vi "Text control 2 v7.1.vi"() -> ()   [LabVIEW 2019]
panel:
  in  "Tab Control":enum32{"Main", "Other parameters"}(tab)
  in  "Plot sample extrema vs time":bool
  out "Line running":i32
  out "Total lines":i32
  out "Path":path=path "C:/users/rlp38/09Apr2009LTtesting/test2.txt"
  out "I vs Vg":cluster{"Y data in":dbl[], "X data in":dbl[]}[](graph)
  out "Is max":dbl format="%.2e"
  out "Id max":dbl format="%.2e"
  out "Ig max":dbl format="%.2e"
  out "Imax vs time":cluster{"Y data in":dbl[], "X data in":dbl[]}[](graph)
  out "Imin vs time":cluster{"Y data in":dbl[], "X data in":dbl[]}[](graph)
  out "I vs Vd":cluster{"Y data in":dbl[], "X data in":dbl[]}[](graph)
  in  "Script":string="#pulsedstressV d 0.03 20 0 0.5 0.0827 5\n#\n#itime m\n#gaterangemode a\n#drainrangemode a\n#pulsed on 0.05 0 0.02\n#transfer d -10 40 1 5 40 35\n#transfer d -10 40 1 5 40 35\n#transfer d -10 40 1 5 40 35\n#output d 0 40 20 0 40 1\n#\n#\n#sample 1 0.008 221 6 0.003\n#samplei 400e-6 200 6 0.002 0.1\n#vsu2pulse -10 4\n#\n#stressV 0.016 0.03 2e-4 0.1e-3 11\n#stressI 220e-7 0.08 15\n#transfer s -1 1 0.5 -0.005 0.005 0.005\n#output s 0 0 0 -0.008 0.008 0.002"
  out "Command running:":string
  out "Serial port data":string
  out "Elapsed Time":dbl caption="Elapsed Time (s)"
  in  "Time Units":u16(ring)=1 items=["Seconds", "Minutes", "Hours"]
  in  "Time Offset":dbl caption="Set Start Time (s)"
  in  "Reset":bool
  in  "Auto Reset":bool
  in  "integration time":u32(slide) max=2 step=1 scale=0.0..2.0
  out "Is on":dbl format="%.2e"
  out "Id on":dbl format="%.2e"
  out "Ig on":dbl format="%.2e"
  out "Ion vs time":cluster{"Y data in":dbl[], "X data in":dbl[]}[](graph)
  out "Ioff vs time":cluster{"Y data in":dbl[], "X data in":dbl[]}[](graph)
  out "Ig min":dbl format="%.2e"
  out "Id min":dbl format="%.2e"
  out "Is min":dbl format="%.2e"
  out "Is off":dbl format="%.2e"
  out "Id off":dbl format="%.2e"
  out "Ig off":dbl format="%.2e"
  in  "Integration time (long)":dbl=0.32 min=0.04 max=2.0 step=0.02 format="%.2f"
  in  "Integration time (short)":dbl=0.0019 min=8e-05 max=0.0019 step=8e-05 format="%^.0e"
  in  "Drain: Compliance":dbl=0.001 format="%.8f"
  in  "Gate: Compliance":dbl=0.001 format="%.8f"
  in  "Interrupt scan":bool
  in  "Interrupt program":bool
  in  "Plot output curve extrema vs time":bool
  in  "Plot transfer curve extrema vs time":bool
  out "I vs time (Bias Stress)":cluster{"Y data in":dbl[], "X data in":dbl[]}[](graph)
  in  "Sample I - Probe 4 (Disabled)":u32(ring)=3 items=["SMU1  ", "SMU2  ", "SMU3  ", "SMU4  ", "SMU5  ", "SMU6  ", "VSU1  ", "VSU2  "]
  in  "Sample I - Source/Common":u32(ring) items=["SMU1  ", "SMU2  ", "SMU3  ", "SMU4  ", "SMU5  ", "SMU6  ", "VSU1  ", "VSU2  "]
  in  "Sample I - Probe 3 (Disabled)":u32(ring)=2 items=["SMU1  ", "SMU2  ", "SMU3  ", "SMU4  ", "SMU5  ", "SMU6  ", "VSU1  ", "VSU2  "]
  in  "Sample I - Drain/Gate":u32(ring)=1 items=["SMU1  ", "SMU2  ", "SMU3  ", "SMU4  ", "SMU5  ", "SMU6  ", "VSU1  ", "VSU2  "]
  in  "Sample - Probe 4":u32(ring)=3 items=["SMU1  ", "SMU2  ", "SMU3  ", "SMU4  ", "SMU5  ", "SMU6  ", "VSU1  ", "VSU2  "]
  in  "Sample - Source/Common":u32(ring) items=["SMU1  ", "SMU2  ", "SMU3  ", "SMU4  ", "SMU5  ", "SMU6  ", "VSU1  ", "VSU2  "]
  in  "Sample - Gate":u32(ring)=2 items=["SMU1  ", "SMU2  ", "SMU3  ", "SMU4  ", "SMU5  ", "SMU6  ", "VSU1  ", "VSU2  "]
  in  "Sample - Drain":u32(ring)=1 items=["SMU1  ", "SMU2  ", "SMU3  ", "SMU4  ", "SMU5  ", "SMU6  ", "VSU1  ", "VSU2  "]
  in  "Gate Range\nmode":u16(ring) items=["Auto", "Limited", "Fixed"]
  in  "Gate Range":u8(slide)=3 max=11 scale=0.0..11.0
  in  "Source/Drain\nRange mode":u16(ring) items=["Auto", "Limited", "Fixed"]
  in  "Source/Drain Range":u8(slide)=3 max=11 scale=0.0..11.0
  in  "Panel Controls":T1={"Emergency Stop"=refnum, "TransGraph Max"=1e-05, "Text/Graph (text=false)"=TRUE} {"TransGraph Max" format="%.2e"}
  in  "Panel Controls 2":T2={"Emergency Stop"=refnum, "TransGraph Max"=1e-05, "Text/Graph (text=false)"=TRUE, "TransGraph Min"=1e-11} {"TransGraph Min" format="%.2e"; "TransGraph Max" format="%.2e"}
  out "error out":errorcluster
  in  "Delay before read (ms)":u32=1000
  in  "byte count":u32=64
  in  "Serial End Mode for Reads":u16(ring)=2 items=["None", "LastBit", "TermChar"]
  in  "Timeout (ms)":u32=10000
  in  "Enable Termination\nChar (T)":bool=TRUE
  in  "Termination char\n(0xA = '\\n' = LF)\n(0xD = '\\r' = CR)":u8=13 format="%.0x"
  in  "flow control":u16(ring) items=["None"=0, "XON/XOFF"=1, "RTS/CTS"=2, "DTR/DSR"=4]
  in  "stop bits":u16(ring)=10 items=["1.0"=10, "1.5"=15, "2.0"=20]
  in  "parity":u16(ring) items=["None", "Odd", "Even", "Mark", "Space"]
  in  "data bits":u16=8 min=5 max=8 step=1
  in  "VISA resource name":refnum<visa-resource-name>="COM6"
  in  "baud rate":u32=9600
  out "Timings Indicator":T3
  in  "Timings (overwritten by the Front Panel)":T4={"integration time"=0, "Short/Long integration time"=0.00064, "hold time (sec)"=0.0, "delay time (sec)"=0.0, "Step Time (0 disables)"=0.0, "sweep method"=0, "Pulse period"=0.005, "Base voltage"=0.0, "Pulse width"=0.0005} {"Pulse width" min=0.0005 max=0.1 step=0.0001 format="%.4f"; "Base voltage" format="%^.4e"; "Pulse period" min=0.005 max=1.0 step=0.0001 format="%.4f"; "sweep method" items=["Continuous", "Pulsed"]; "Step Time (0 disables)" format="%.2f"; "delay time (sec)" format="%.4f"; "hold time (sec)" format="%.4f"; "Short/Long integration time" format="%^.0e"; "integration time" scale=0.0..2.0}
  in  "Probe 4":cluster{"on/off":bool, "Voltage":dbl} {"Voltage" min=-100.0 max=100.0 format="%.2f"}
  in  "Full Reset":bool
  in  "Standby":T5
  out "Probe 4 Indicator":cluster{"on/off":bool, "Voltage":dbl} {"Voltage" min=-100.0 max=100.0 format="%.2f"}
  in  "Transfer/Output - Drain":u32(ring)=1 items=["SMU1  ", "SMU2  ", "SMU3  ", "SMU4  ", "SMU5  ", "SMU6  ", "VSU1  ", "VSU2  "]
  in  "Transfer/Output - Gate":u32(ring)=2 items=["SMU1  ", "SMU2  ", "SMU3  ", "SMU4  ", "SMU5  ", "SMU6  ", "VSU1  ", "VSU2  "]
  in  "Transfer/Output - Source/Common":u32(ring) items=["SMU1  ", "SMU2  ", "SMU3  ", "SMU4  ", "SMU5  ", "SMU6  ", "VSU1  ", "VSU2  "]
  in  "Transfer/Output - Probe 4":u32(ring)=3 items=["SMU1  ", "SMU2  ", "SMU3  ", "SMU4  ", "SMU5  ", "SMU6  ", "VSU1  ", "VSU2  "]
  in  "Pulsed Stress V - Probe 4":u32(ring)=3 items=["SMU1  ", "SMU2  ", "SMU3  ", "SMU4  ", "SMU5  ", "SMU6  ", "VSU1  ", "VSU2  "]
  in  "Pulsed Stress V - Vextra":u32(ring)=6 items=["SMU1  ", "SMU2  ", "SMU3  ", "SMU4  ", "SMU5  ", "SMU6  ", "VSU1  ", "VSU2  "]
  in  "Pulsed Stress V - Drain":u32(ring)=1 items=["SMU1  ", "SMU2  ", "SMU3  ", "SMU4  ", "SMU5  ", "SMU6  ", "VSU1  ", "VSU2  "]
  in  "Pulsed Stress V - Source/Common":u32(ring) items=["SMU1  ", "SMU2  ", "SMU3  ", "SMU4  ", "SMU5  ", "SMU6  ", "VSU1  ", "VSU2  "]
  in  "Pulsed Stress V - Gate":u32(ring)=2 items=["SMU1  ", "SMU2  ", "SMU3  ", "SMU4  ", "SMU5  ", "SMU6  ", "VSU1  ", "VSU2  "]
  in  "FPP - Drain":u32(ring)=1 items=["SMU1  ", "SMU2  ", "SMU3  ", "SMU4  ", "SMU5  ", "SMU6  ", "VSU1  ", "VSU2  "]
  in  "FPP - Gate":u32(ring)=2 items=["SMU1  ", "SMU2  ", "SMU3  ", "SMU4  ", "SMU5  ", "SMU6  ", "VSU1  ", "VSU2  "]
  in  "FPP - Probe 1":u32(ring) items=["SMU1  ", "SMU2  ", "SMU3  ", "SMU4  ", "SMU5  ", "SMU6  ", "VSU1  ", "VSU2  "]
  in  "FPP - Probe 2":u32(ring)=3 items=["SMU1  ", "SMU2  ", "SMU3  ", "SMU4  ", "SMU5  ", "SMU6  ", "VSU1  ", "VSU2  "]
  in  "FPP - Source":u32(ring)=6 items=["SMU1  ", "SMU2  ", "SMU3  ", "SMU4  ", "SMU5  ", "SMU6  ", "VSU1  ", "VSU2  "]
  in  "Stress V - Drain":u32(ring)=1 items=["SMU1  ", "SMU2  ", "SMU3  ", "SMU4  ", "SMU5  ", "SMU6  ", "VSU1  ", "VSU2  "]
  in  "Stress V - Gate":u32(ring)=2 items=["SMU1  ", "SMU2  ", "SMU3  ", "SMU4  ", "SMU5  ", "SMU6  ", "VSU1  ", "VSU2  "]
  in  "Stress V - Source/Common":u32(ring) items=["SMU1  ", "SMU2  ", "SMU3  ", "SMU4  ", "SMU5  ", "SMU6  ", "VSU1  ", "VSU2  "]
  in  "Stress I - Drain/Gate":u32(ring)=1 items=["SMU1  ", "SMU2  ", "SMU3  ", "SMU4  ", "SMU5  ", "SMU6  ", "VSU1  ", "VSU2  "]
  in  "Stress I - Source/Common":u32(ring) items=["SMU1  ", "SMU2  ", "SMU3  ", "SMU4  ", "SMU5  ", "SMU6  ", "VSU1  ", "VSU2  "]
  in  "VSU2 Stress - Source/Common":u32(ring) items=["SMU1  ", "SMU2  ", "SMU3  ", "SMU4  ", "SMU5  ", "SMU6  ", "VSU1  "]
  in  "VISA resource name in":refnum<visa-resource-name>="GPIB0::14::INSTR"
  in  "Gate":T6={"Gate Start"=0.0, "Gate Stop"=2.0, "Gate Step (linear only)"=1.0, "Gate Compliance"=0.0001, "Gate PComp"=0.0, "Range mode"=0, "Range"=6} {"Range" max=11 scale=0.0..11.0; "Range mode" items=["Auto", "Limited", "Fixed"]; "Gate PComp" format="%^.2e"; "Gate Compliance" format="%^.2e"; "Gate Step (linear only)" format="%^.4e"; "Gate Stop" format="%^.4e"; "Gate Start" format="%^.4e"}
  in  "Drain 2":T7={"Drain Start"=0.0, "Drain Stop"=2.0, "Drain Compliance"=0.0001, "Drain Step"=1.0, "Drain PComp"=0.0, "Range mode"=0, "Range"=6} {"Range" max=11 scale=0.0..11.0; "Range mode" items=["Auto", "Limited", "Fixed"]; "Drain PComp" format="%^.2e"; "Drain Step" format="%^.4e"; "Drain Compliance" format="%^.2e"; "Drain Stop" format="%^.4e"; "Drain Start" format="%^.4e"}
  # "Time"
  # "Syntax:\nitime [s|m|l] time(sec): [s|m|l] determines the integration time setting (small|medium|long) and time sets the value.\nNOTE: The value of the integration time has to be within the range allowed by its category (s|m|l), otherwise, the closest value will be used. (e.g. if the category is set to short but the time value is very long, the actual value used will be the maximum short integration time.\nIntegration times:\n    Short: Default: 640 us. Range: 8E-5 - 1.92E-3 seconds.\n    Medium: Fixed at 1 NPL cycle (0.02 seconds).\n    Long: Default: 16 NPL cycles (0.32 seconds). Range: 2-100 NPL cycles (0.04 seconds - 2 seconds).\ngaterangemode [a|l|f]\ndrainrangemode [a|l|f]\npulsed [on|off] PulsePeriod(sec) PulseBaseVoltage PulseONWidth(sec)\nstandby [on l off]\nwait NumMilliseconds\nwait-min NumMinutes\n# texthere = comment\nProbe4 [ON|OFF] Voltage\ntransfer [s|d] VgStart VgStop VgStep VdStart VdStop VdStep\noutput [s|d] VgStart VgStop VgStep VdStart VdStop VdStep\nsample Vg Vd NumSamples Time(s) SampleInterval(s)\nsamplei Idg NumSamples Time(s) SampleInterval(s) VDGcompliance\n100 samples is approximately 13 seconds with medium integration\n# if in doubt use SampleInterval(s) = 0.004\n    NOTE: When doing bias stress measurements, it is best to set the Time Units to \"Seconds\", as the \"sample\" command has been configured to give the output to seconds.\nstressV VG VD IGcompliance IDcompliance Duration(sec)\nstressI IDG VDGcompliance Duration(sec)\nvsu2pulse Bias Duration(s)\npulsedstressV [s|d] VEstop VgON VgOFF Period(s) PulseONwidth(s) Vd\nsample-fpp Vg Vd NumSamples Time\nresample-fpp Vg Vd\ntransfer-fpp [s|d] VgStart VgStop VgStep VdStart VdStop VdStep\noutput-fpp [s|d] VgStart VgStop VgStep VdStart VdStop VdStep\nserial SerialPortCommand"
  # "1\n2\n3\n4\n5\n6\n7\n8\n9\n10\n11\n12\n13\n14\n15\n16\n17\n18\n19\n20"
  # "SMUs"
  # "Serial port settings"
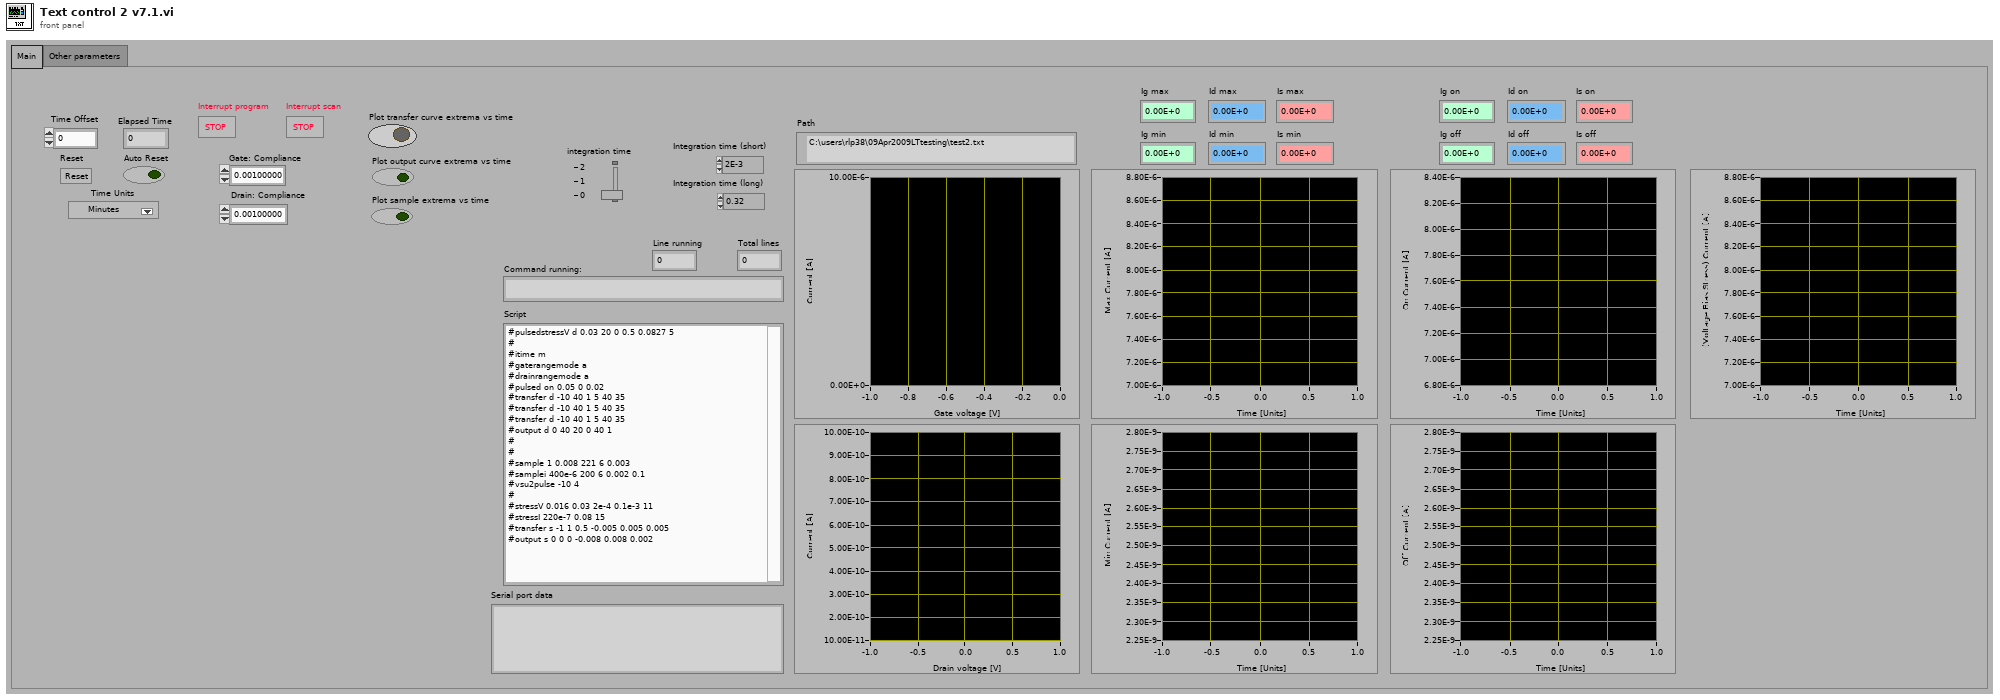
[diagram p1: front panel]
types:
  T1 = cluster{"Emergency Stop":refnum<vi>, "TransGraph Max":dbl, "Text/Graph (text=false)":bool}
  T2 = cluster{"Emergency Stop":refnum<vi>, "TransGraph Max":dbl, "Text/Graph (text=false)":bool, "TransGraph Min":dbl}
  T3 = cluster{"integration time (0:s, 1:m, 2:l)":u32, "Short/Long integration time":dbl, "hold time (sec)":dbl, "delay time (sec)":dbl, "Step Time (0 disables)":dbl, "sweep method":u16, "Pulse period":dbl, "Base voltage":dbl, "Pulse width":dbl}
  T4 = cluster{"integration time":u32, "Short/Long integration time":dbl, "hold time (sec)":dbl, "delay time (sec)":dbl, "Step Time (0 disables)":dbl, "sweep method":u16, "Pulse period":dbl, "Base voltage":dbl, "Pulse width":dbl}
  T5 = cluster{"Gate Standby":bool, "Drain Standby":bool}
  T6 = cluster{"Gate Start":dbl, "Gate Stop":dbl, "Gate Step (linear only)":dbl, "Gate Compliance":dbl, "Gate PComp":dbl, "Range mode":u16, "Range":u8}
  T7 = cluster{"Drain Start":dbl, "Drain Stop":dbl, "Drain Compliance":dbl, "Drain Step":dbl, "Drain PComp":dbl, "Range mode":u16, "Range":u8}
  T8 = enum16{"open", "replace", "create", "open or create", "replace or create", "replace or create with confirmation"}
  T9 = cluster{"V2 Start":dbl, "V2 Step":dbl, "Number of points":i32}
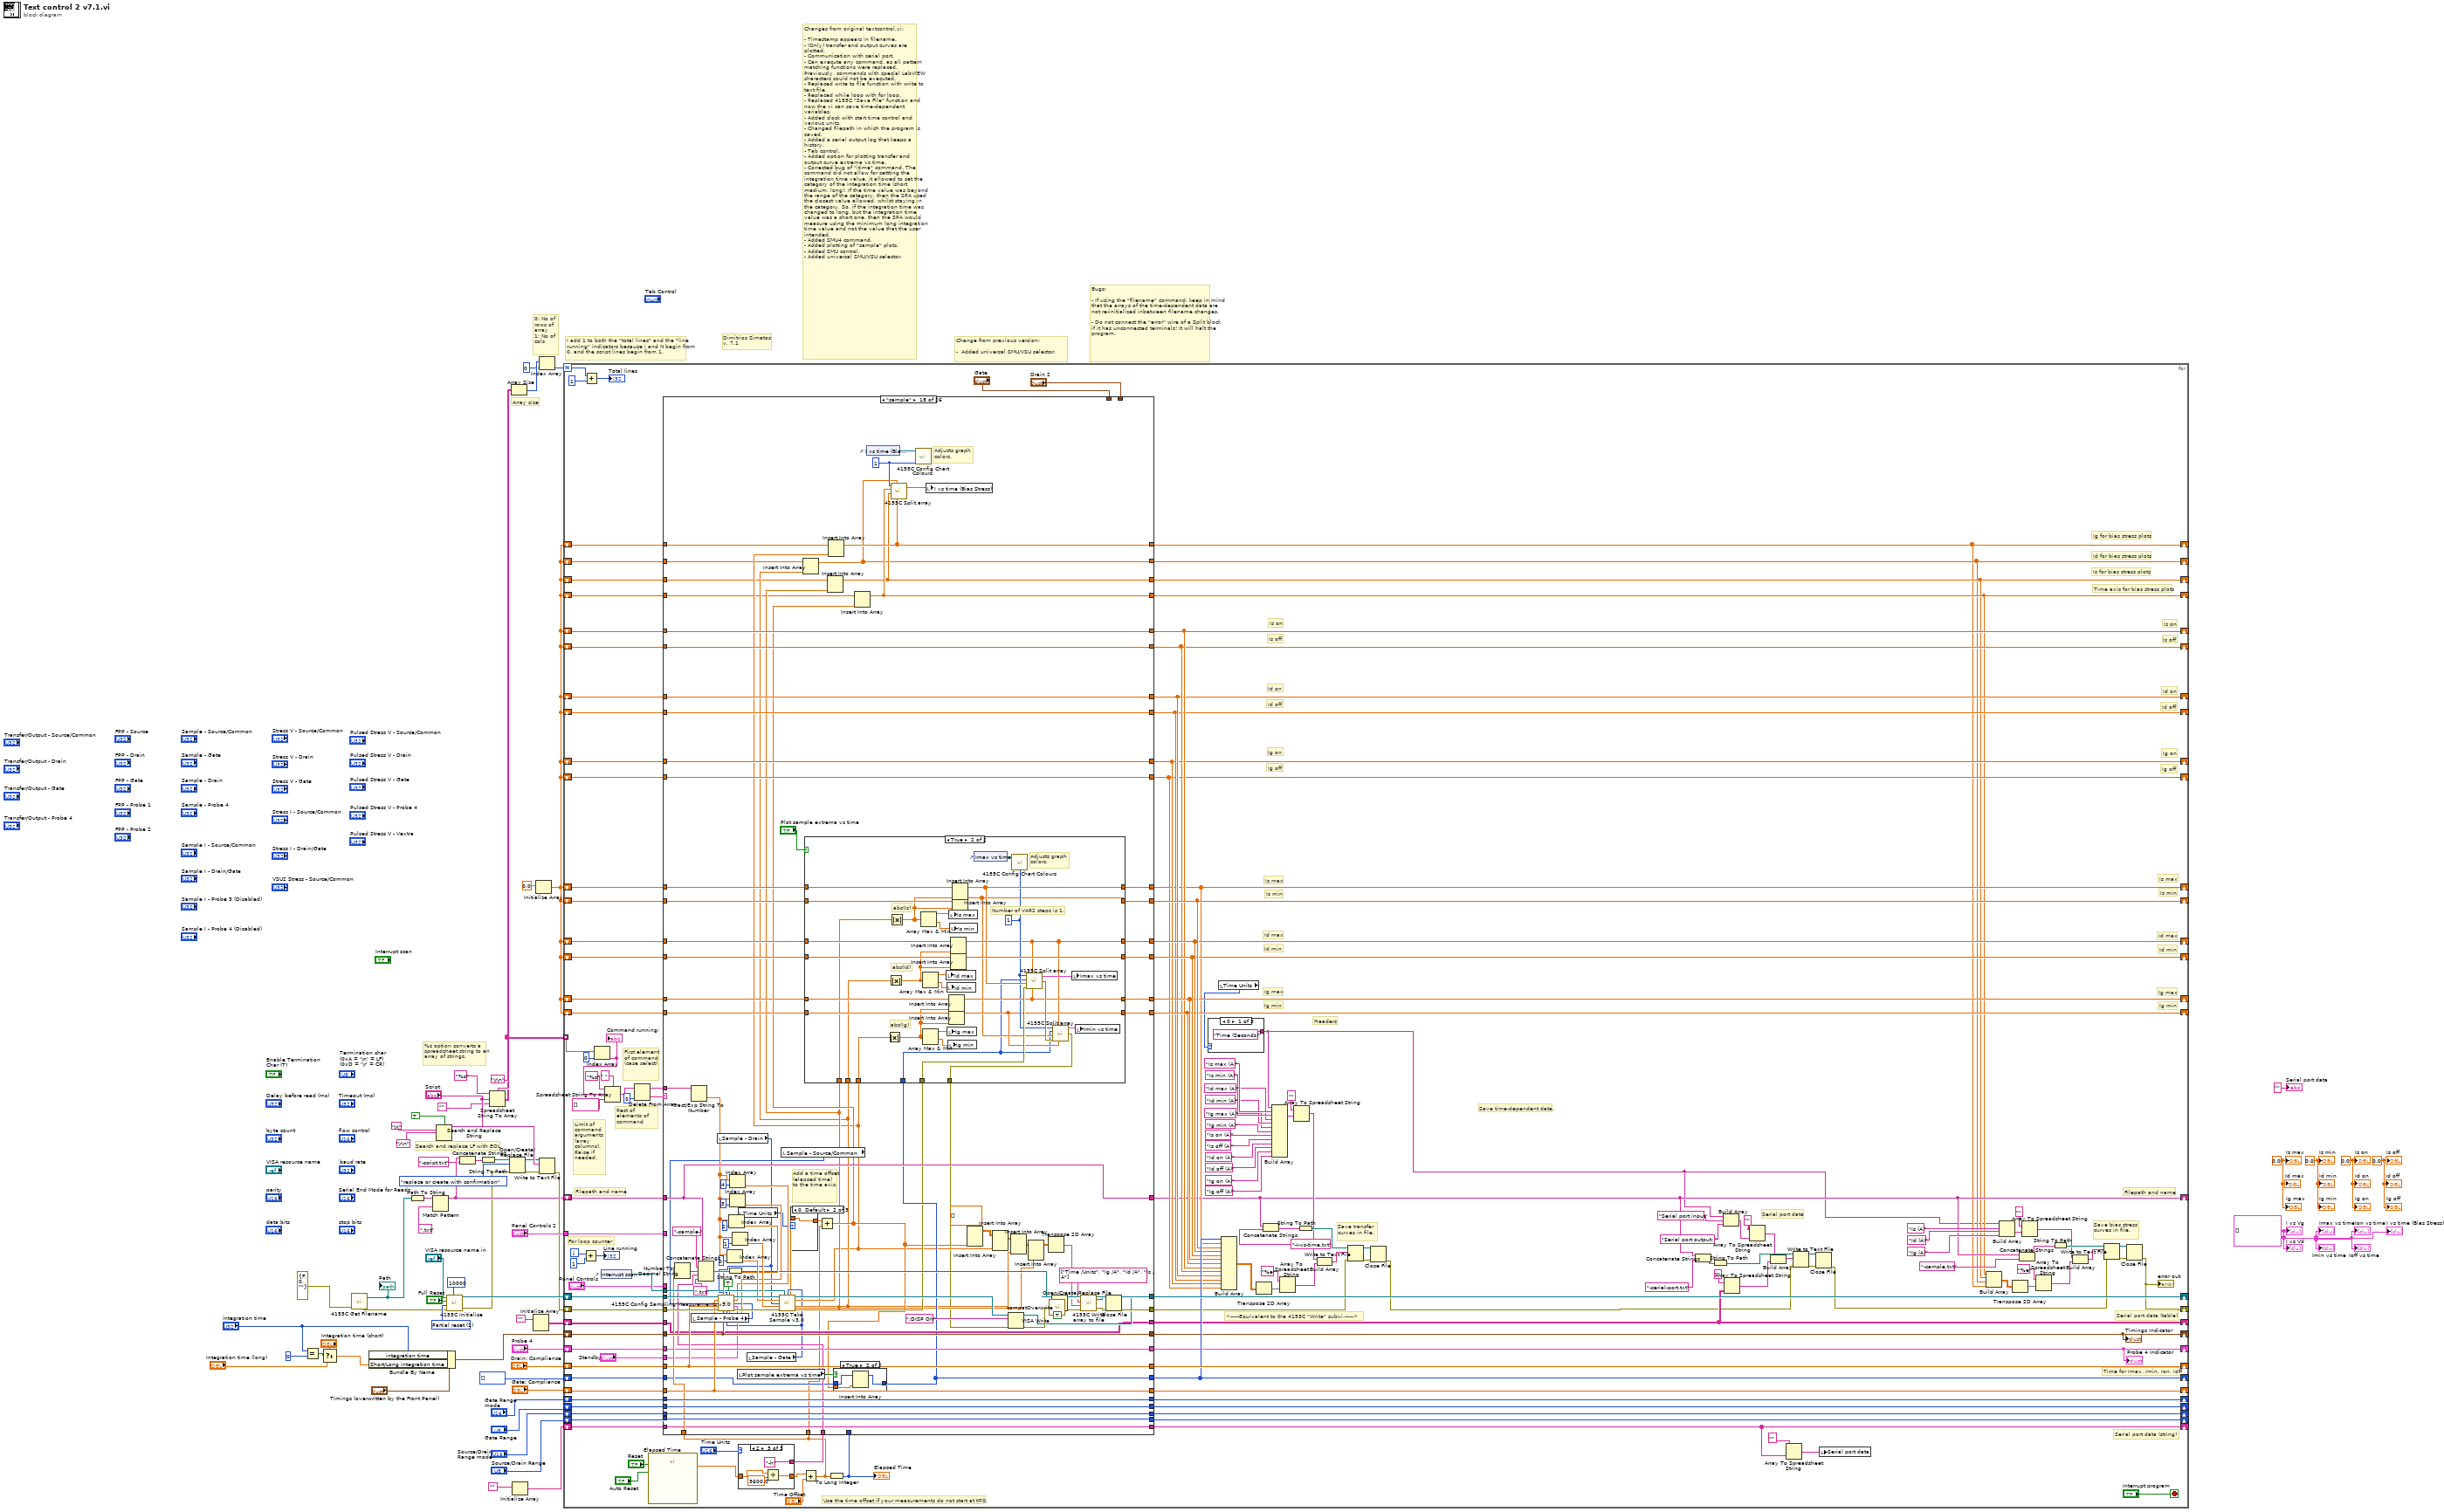
[diagram p0: block diagram]
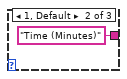
[diagram p2: hidden frame]
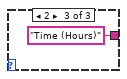
[diagram p3: hidden frame]
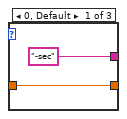
[diagram p4: hidden frame]
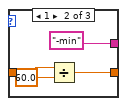
[diagram p5: hidden frame]
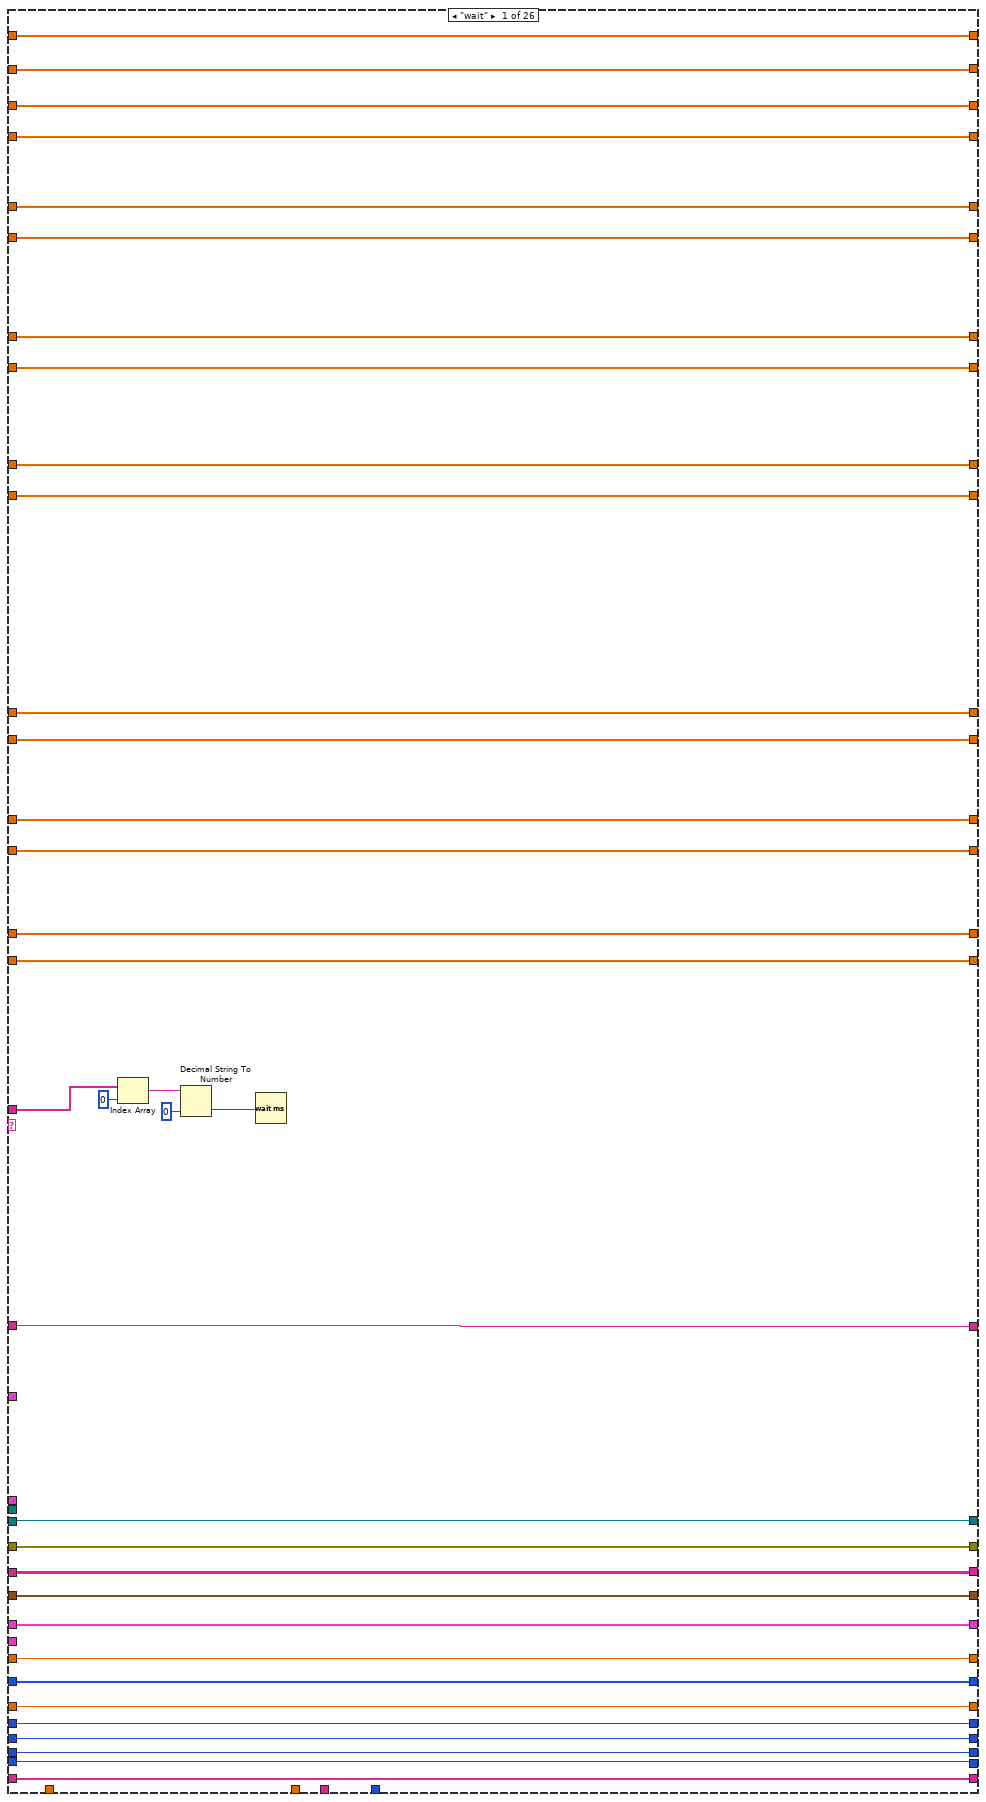
[diagram p6: hidden frame]
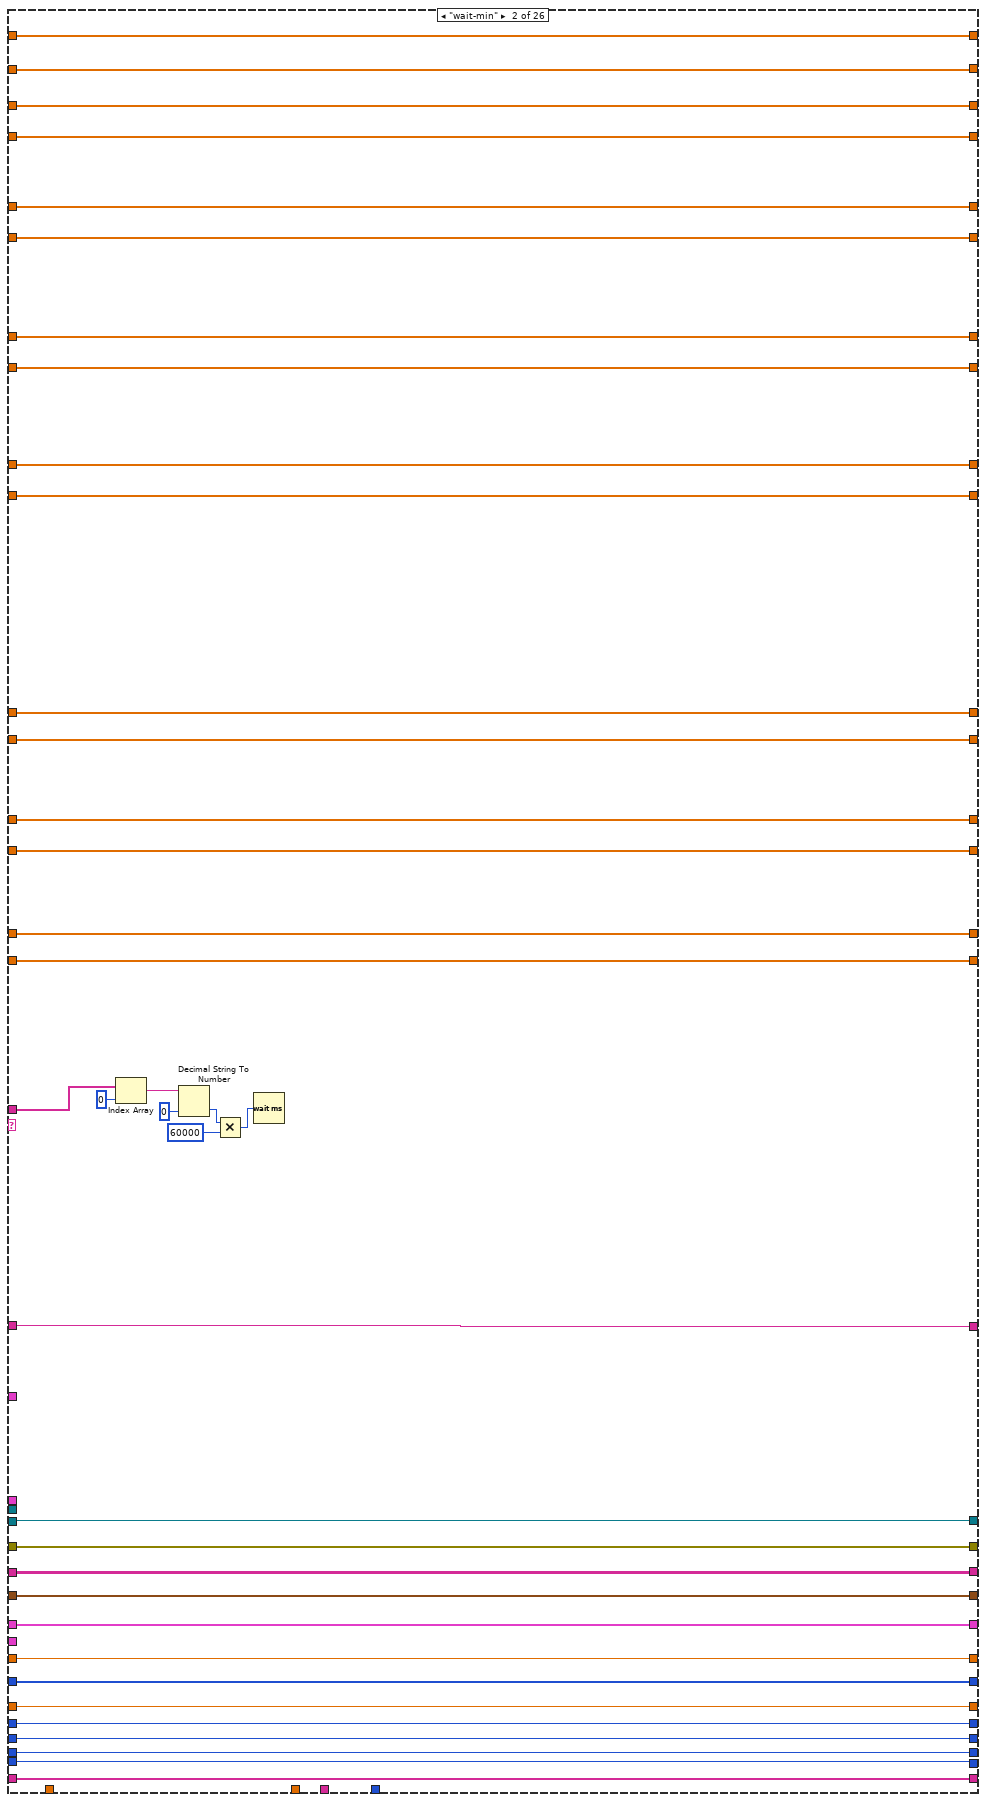
[diagram p7: hidden frame]
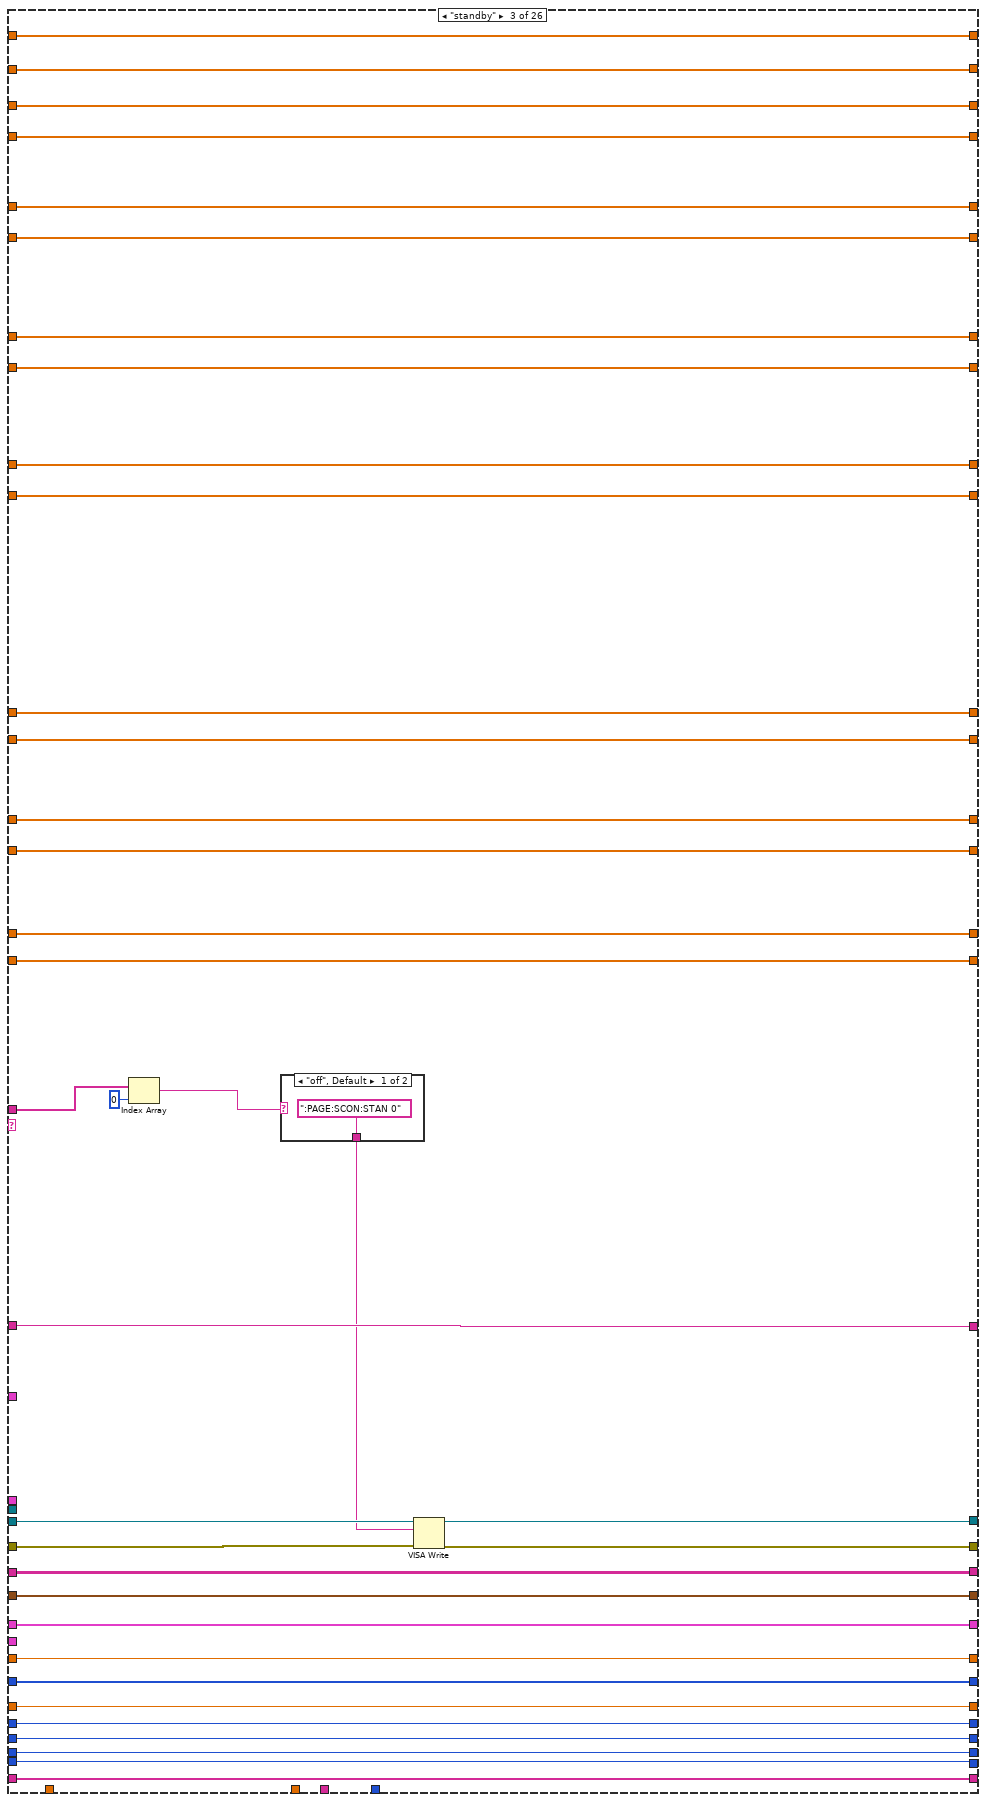
[diagram p8: hidden frame]
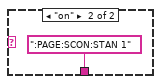
[diagram p9: hidden frame]
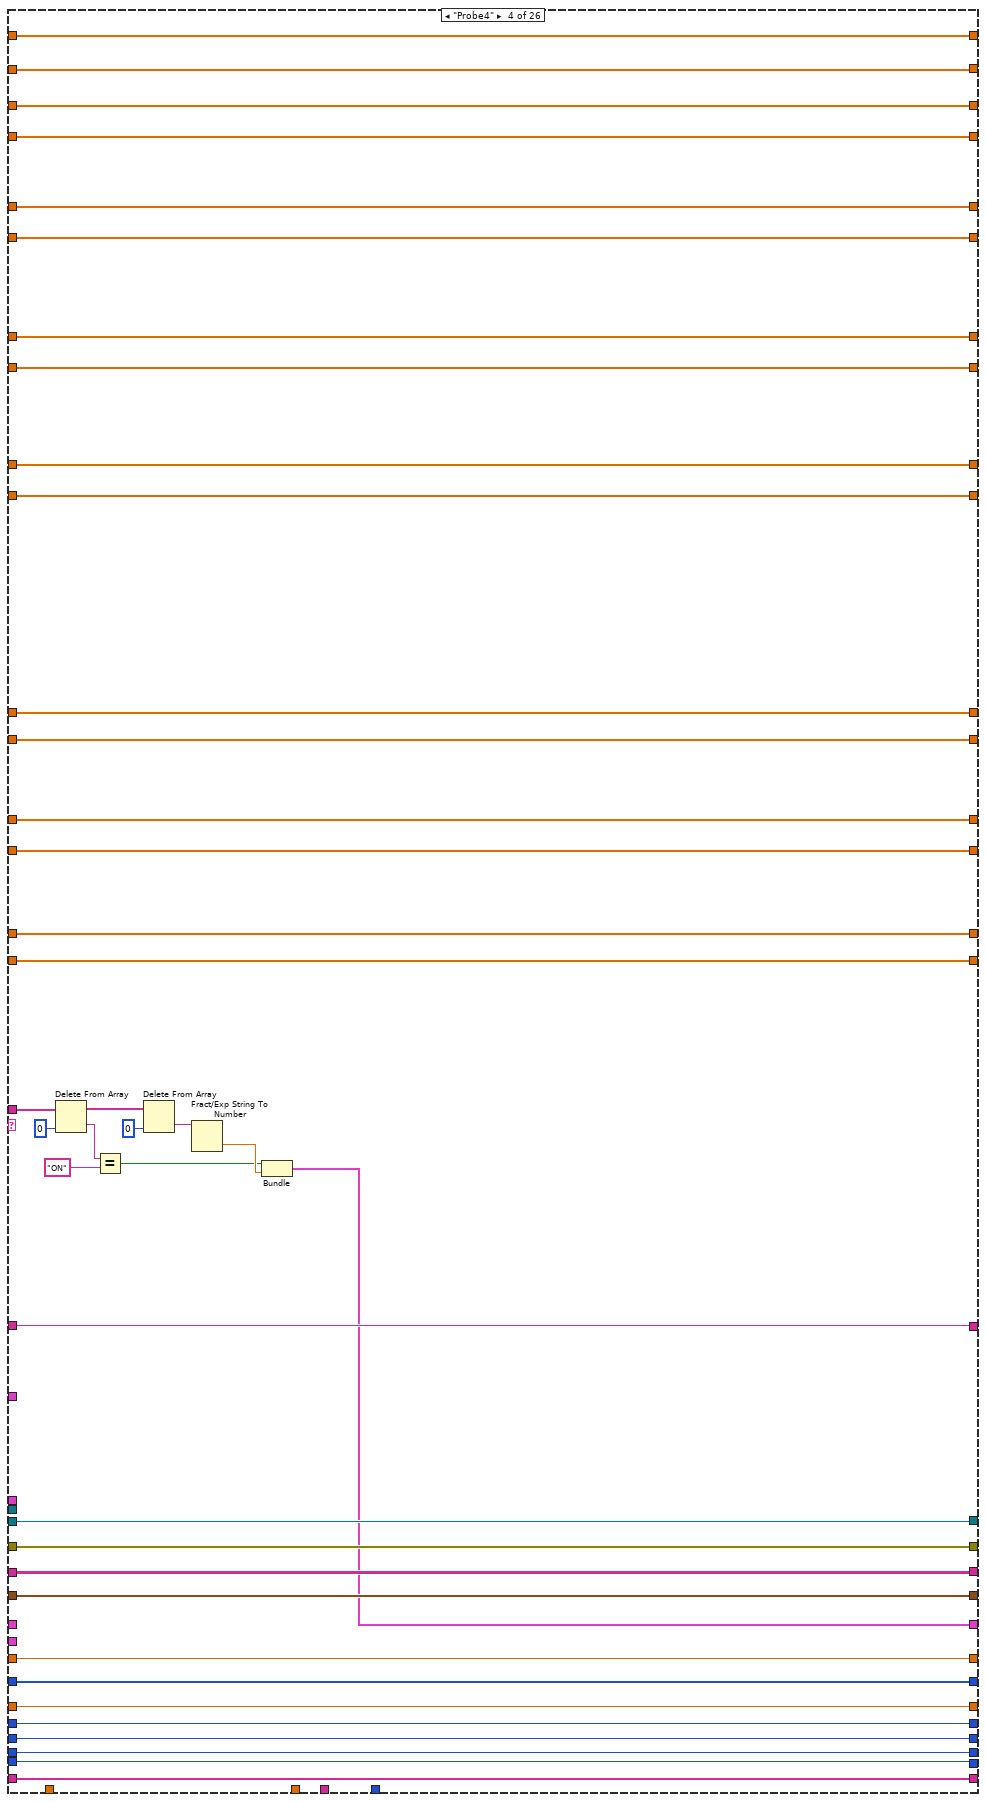
[diagram p10: hidden frame]
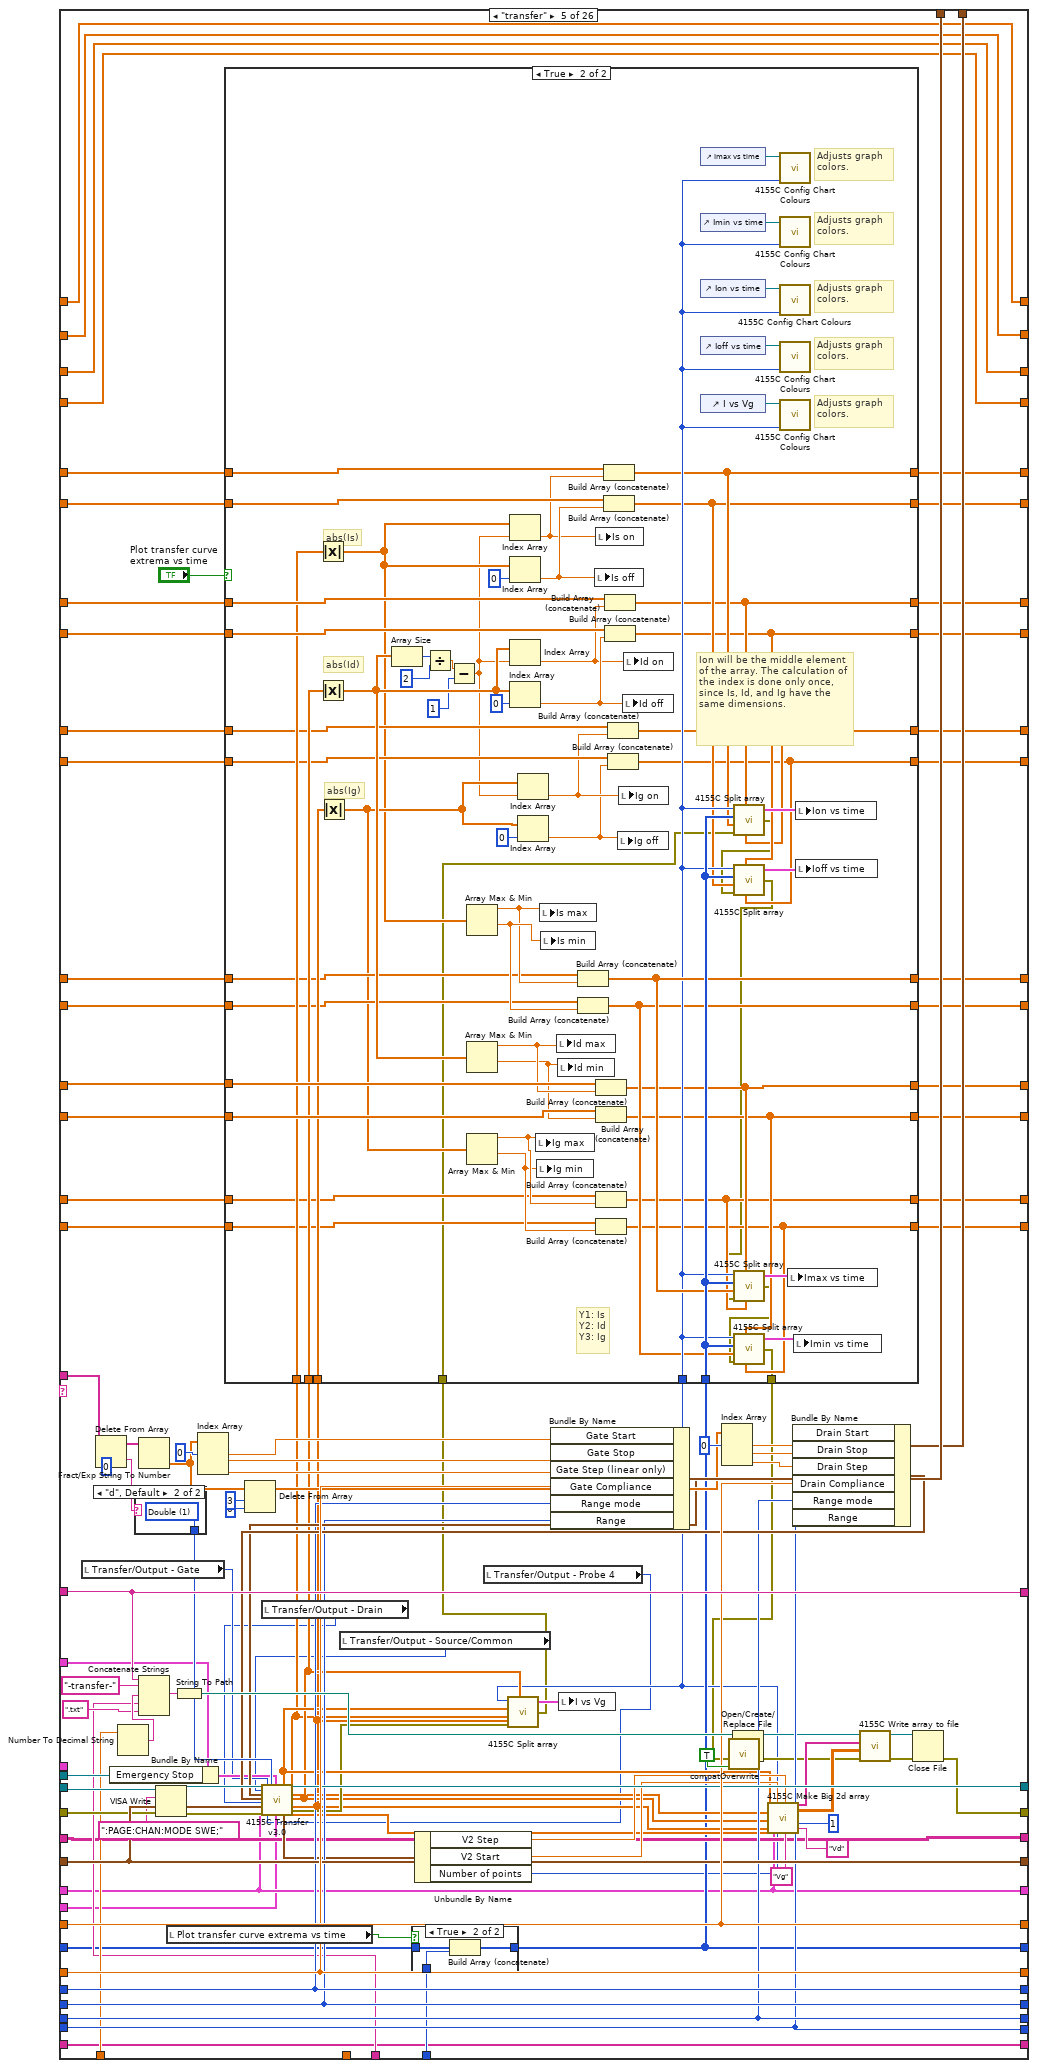
[diagram p11: hidden frame]
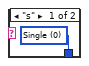
[diagram p14: hidden frame]
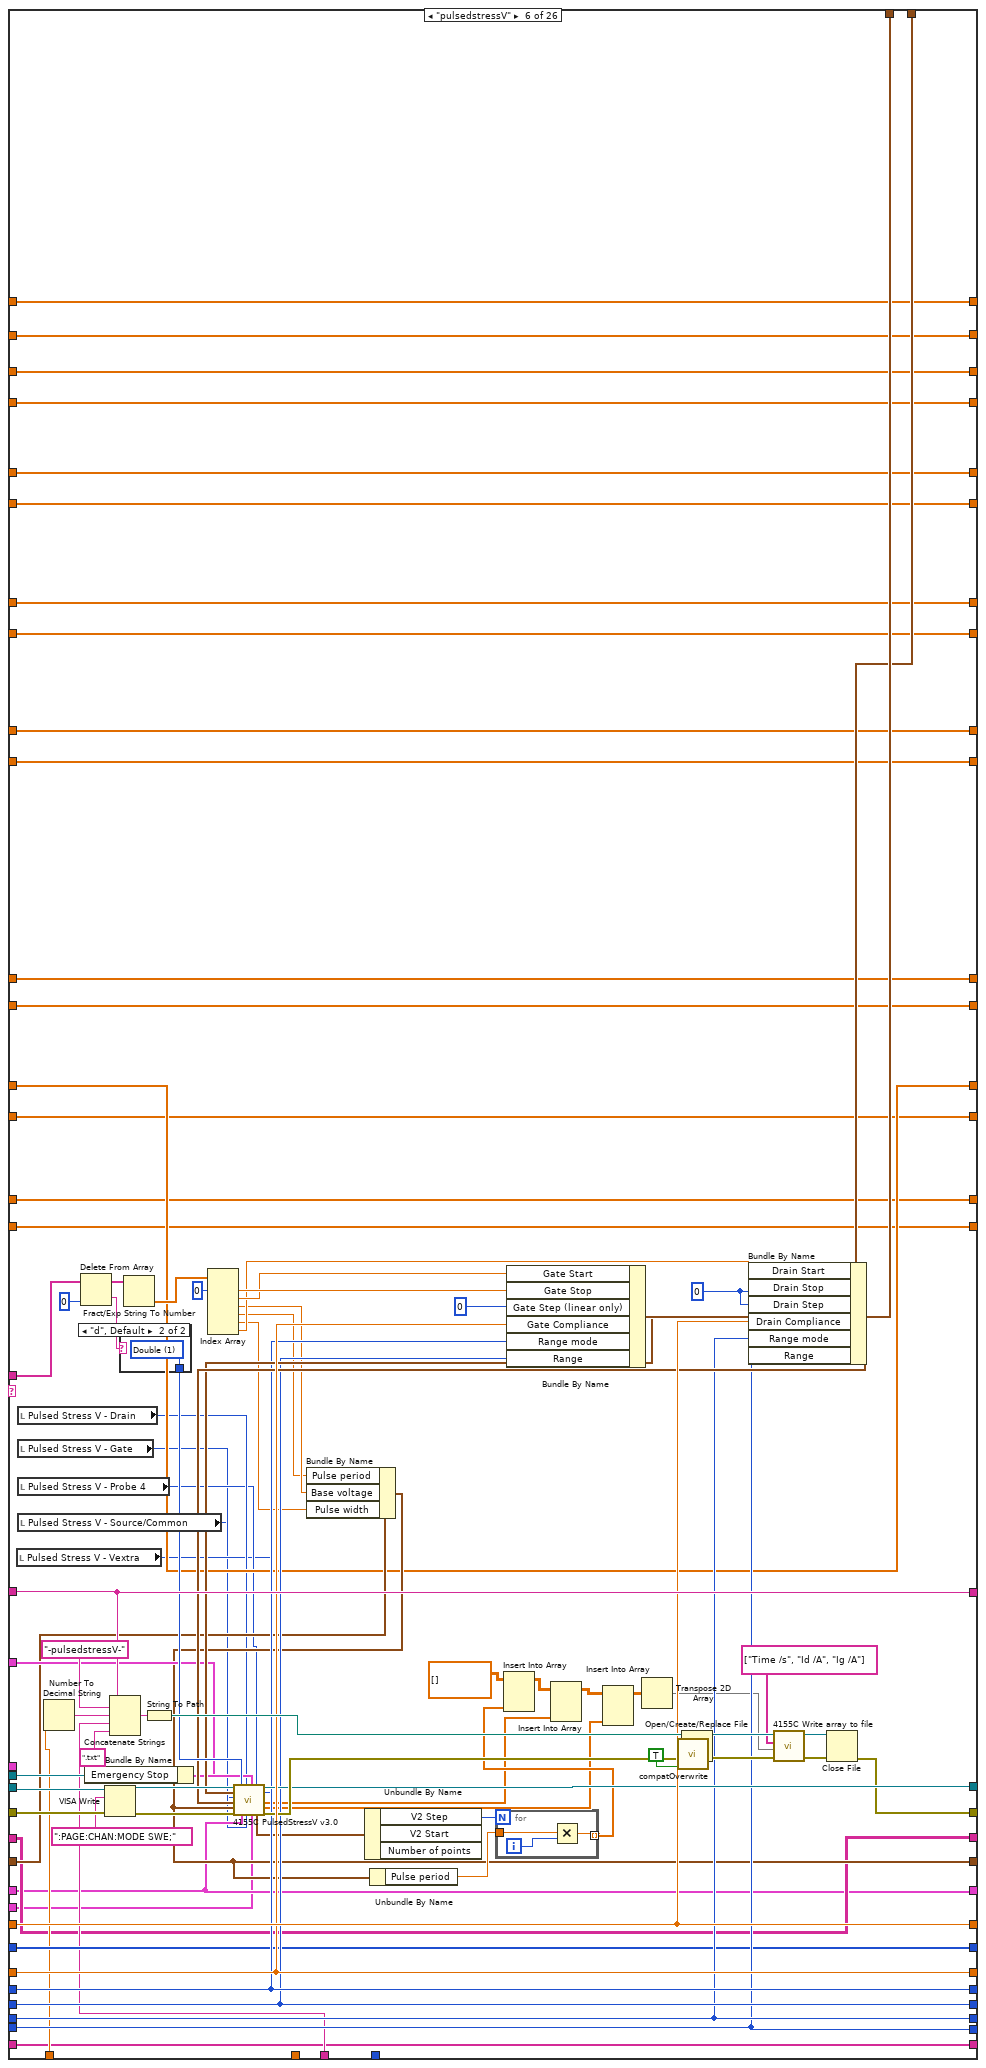
[diagram p15: hidden frame]
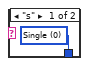
[diagram p16: hidden frame]
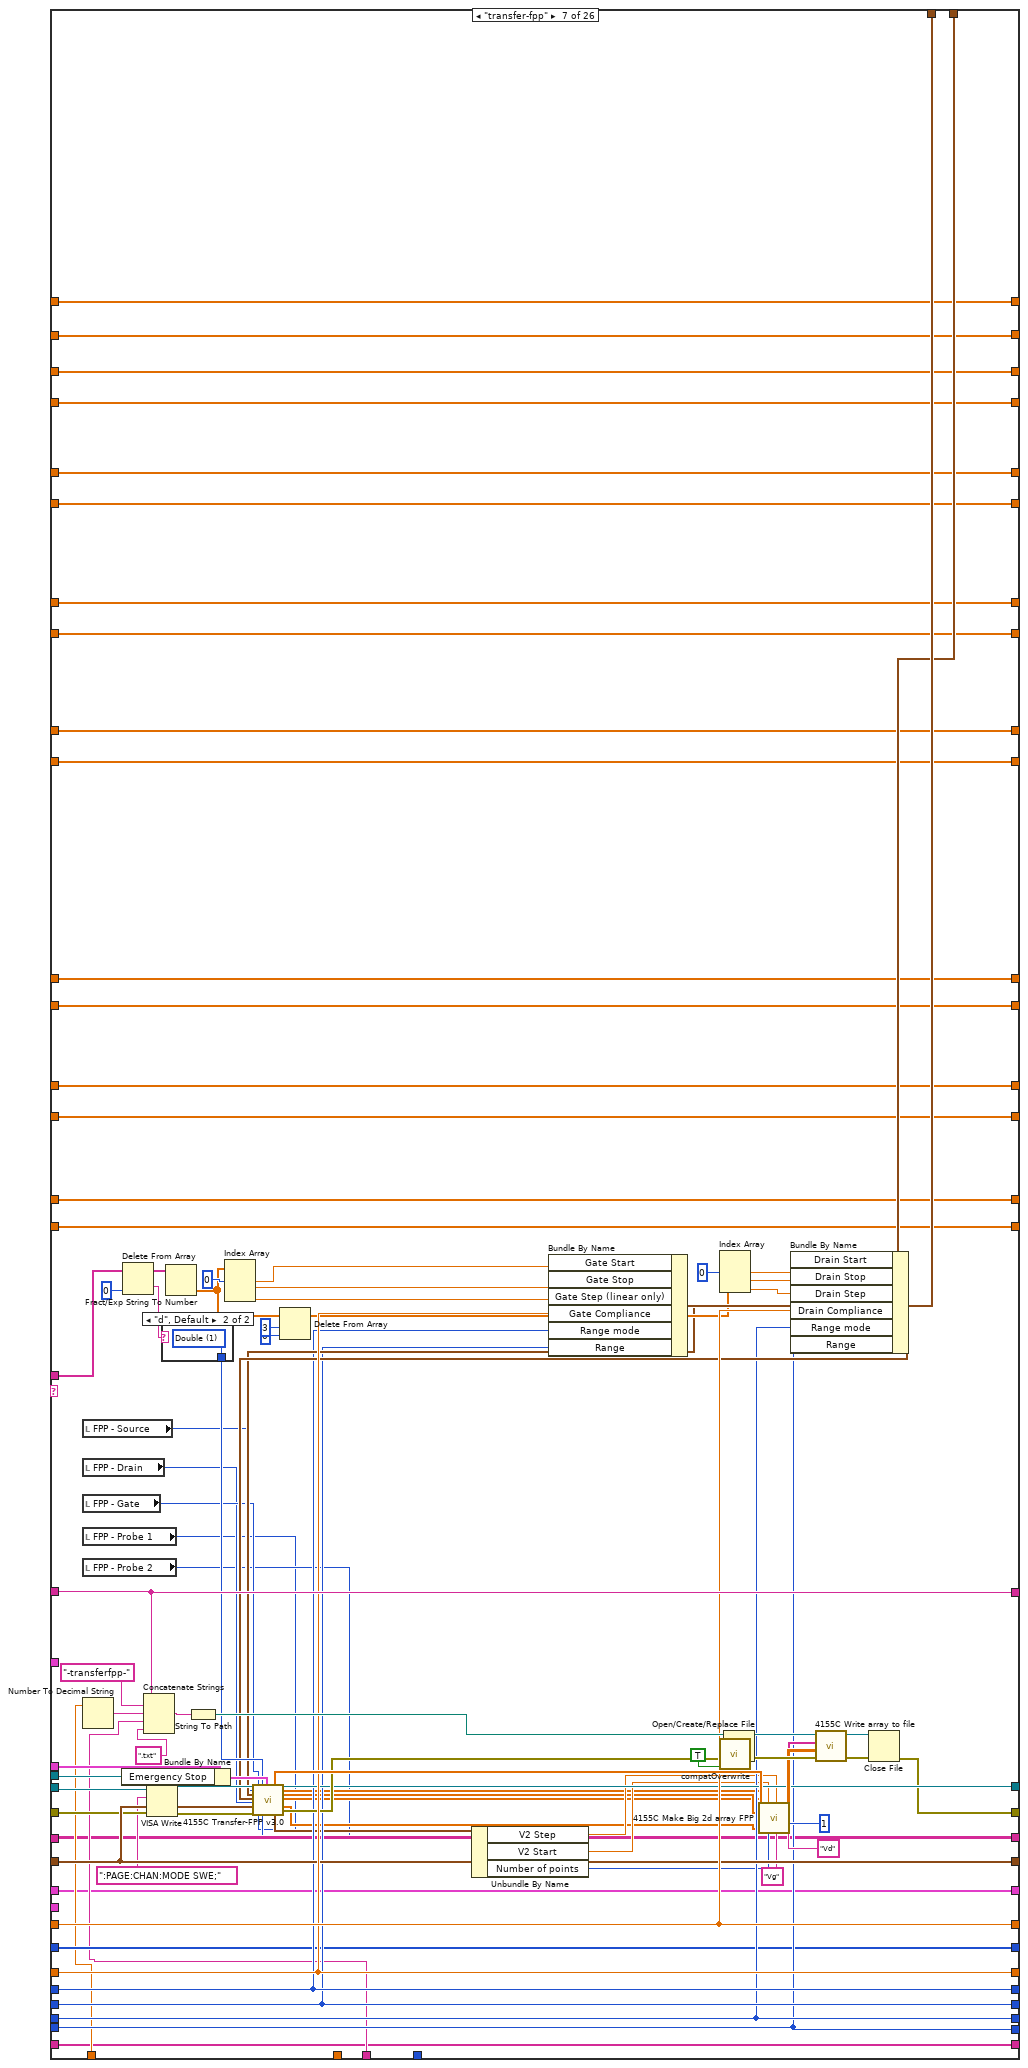
[diagram p17: hidden frame]
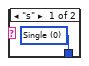
[diagram p18: hidden frame]
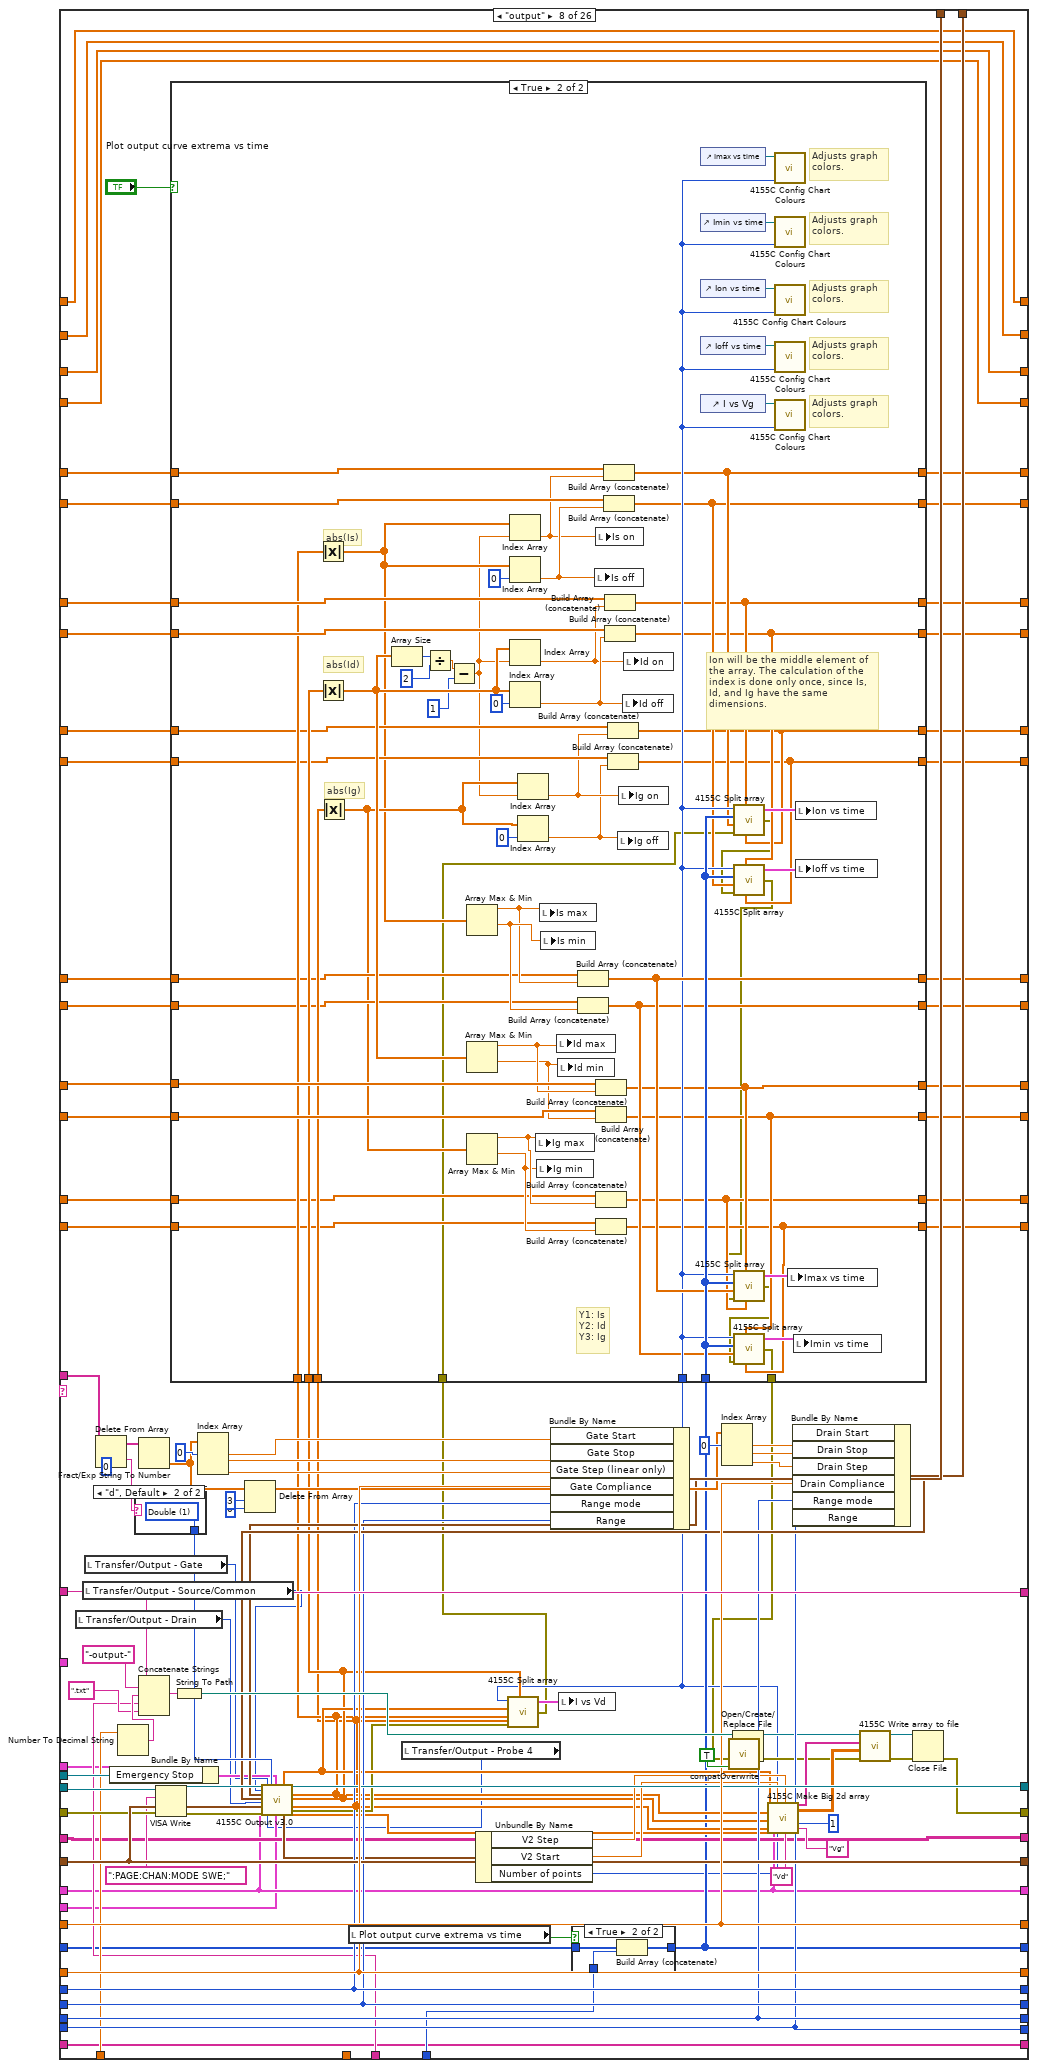
[diagram p19: hidden frame]
diagram:
  w2 = cluster{"Y data in":dbl[], "X data in":dbl[]}[] [] ("I vs Vg")
  w9 = 0.0 ("Is off")
  w10 = 0.0 ("Is on")
  w11 = 0.0 ("Is min")
  w12 = 0.0 ("Is max")
  w55 = u16 1 items=["Reset All", "Partial reset"] ("Type of reset")
  # "Change from previous version:\n\n-  Added universal SMU/VSU selector."
  # "I add 1 to both the \"total lines\" and the \"line running\" indicators because i and N begin from 0, and the script lines begin from 1."
  # "Bugs:\n\n- If using the \"filename\" command, keep in mind that the arrays of the time-dependent data are not re-initialized inbetween filename changes. \n\n- Do not connect the \"error\" wire of a Split block if it has unconnected terminals! It will halt the program."
  # "Array size"
  # "%s option converts a spreadsheet string to an array of strings."
  # "0: No of rows of array\n1: No of cols"
  # "Dimitrios Simatos\nv. 7.1"
  # "Changes from original textcontrol.vi:\n\n- Timestamp appears in filename.\n- (Only) transfer and output curves are plotted.\n- Communication with serial port.\n- Can execute any command, as all pattern matching functions were replaced. Previously, commands with special LabVIEW characters could not be executed.\n- Replaced write to file function with write to text file.\n- Replaced while loop with for loop.\n- Replaced 4155C \"Save File\" function and now the vi can save time-dependent variables.\n- Added clock with start time control and various units.\n- Changed filepath in which the program is saved.\n- Added a serial output log that keeps a history.\n- Tab control.\n- Added option for plotting transfer and output curve extrema vs time.\n- Corrected bug of \"itime\" command. The command did not allow for settting the integration time value, it allowed to set the category of the integration time (short, medium, long). If the time value was beyond the range of the category, then the SPA used the closest value allowed, whilst staying in the category. So, if the integration time was changed to long, but the integration time value was a short one, then the SPA would measure using the minimum long integration time value and not the value that the user intended.\n- Added SMU4 command.\n- Added plotting of \"sample\" plots.\n- Added SMU control.\n- Added universal SMU/VSU selector."
  # "Search and replace LF with EOL"
  n1 = Equal?(x="integration time", y=u32 0) -> (x = y?=w56:bool)
  n2 = Select(t="Integration time (short)", s=w56, f="Integration time (long)") -> (s? t:f=w17:dbl)
  n3 = call "4155C Get Filename.vi"("error in (no error)"=errorcluster {"status"=FALSE, "code"=0, "source"=""}) -> ("error out"=w50:errorcluster, "path"=w25:path)  [unwired: 2 in, 1 out]
  "Path" <- w25
  n4 = Bundle By Name(cluster="Timings (overwritten by the Front Panel)", "integration time"="integration time", "Short/Long integration time"=w17) -> (w48:T4)
  n5 = Path To String(path=w25) -> (string=w26:string)
  n6 = Match Pattern(string=w26, regular expression=".txt") -> (before substring=w15:string)  [unwired: 1 in, 3 out]
  n7 = Search and Replace String(replace all?=TRUE ("replace all? (F)"), input string="Script", search string="\n", replace string="\r\n") -> (result string=w38:string)  [unwired: 4 in, 3 out]
  n8 = call "4155C Initialise.vi"("VISA resource name in"="VISA resource name in", "Reset"="Full Reset", "Type of reset"=w55, "error in (no error)"=w50, "VISA Timeout Value"=u32 10000) -> ("VISA Resource Name out"=w49:refnum<visa-resource-name>, "error out"=w7:errorcluster)
  n9 = Concatenate Strings(w15, "-script.txt" ("string")) -> (w16:string)
  n10 = String To Path(string=w16) -> (path=w5:path)
  n11 = Spreadsheet String To Array(delimiter (Tab)="\r\n", format string="%s", spreadsheet string="Script", array type (2D Dbl)="") -> (array=w29:string[][])
  n12 = Open/Create/Replace File(file path (use dialog)=w5, error in=w7, operation (0:open)=T8."replace or create with confirmation") -> (refnum out=w4:refnum<file>, error out=w6:errorcluster)  [unwired: 3 in, 1 out]
  n13 = Array Size(array=w29) -> (size(s)=w33:i32[])
  n14 = Initialize Array("") -> (w20:string[])  [unwired: 1 in]
  n15 = Initialize Array("") -> (w18:string[][])  [unwired: 2 in]
  n16 = Initialize Array(0.0 ("element")) -> (w1:dbl[])  [unwired: 1 in]
  n17 = Index Array(array=w33, index=0) -> (element=w31:i32)
  n18 = Write to Text File(file (use dialog)=w4, text=w38, error in=w6) -> (error out=w23:errorcluster)  [unwired: 1 in, 2 out]
  n19 = for {
    N: w31 -> [w157]
    shift-left: "Source/Drain Range" -> [w197]
    shift-right: [w193] -> _
    shift-left: "Source/Drain\nRange mode" -> [w198]
    shift-right: [w194] -> _
    shift-left: "Gate Range" -> [w199]
    shift-right: [w195] -> _
    shift-left: "Gate Range\nmode" -> [w200]
    shift-right: [w196] -> _
    shift-left: "Gate: Compliance" -> [w208]
    shift-right: [w205] -> _
    shift-left: "Drain: Compliance" -> [w209]
    shift-right: [w206] -> _
    shift-left: w48 -> [w210]
    shift-right: [w62] -> _
    shift-left: w23 -> [w211]
    shift-right: [w63] -> _
    shift-left: w49 -> [w212]
    shift-right: [w207] -> _
    shift-left: w15 -> [w213]
    shift-right: [w70] -> _
    tunnel: "Panel Controls 2" -> [w191]
    shift-right: [w110] -> _
    shift-left: w1 -> [w190]
    shift-right: [w144] -> _
    shift-left: i32[] [] -> [w186]
    tunnel: w29 -> [w185] mode=indexing
    shift-right: [w109] -> _
    shift-left: w1 -> [w162]
    shift-right: [w139] -> _
    shift-left: w20 -> [w149]
    shift-right: [w140] -> _
    shift-left: w18 -> [w142]
    shift-right: [w103] -> _
    shift-left: w1 -> [w131]
    shift-right: [w104] -> _
    shift-left: w1 -> [w130]
    shift-right: [w108] -> _
    shift-left: w1 -> [w119]
    shift-right: [w107] -> _
    shift-left: w1 -> [w118]
    shift-right: [w101] -> _
    shift-left: w1 -> [w117]
    shift-right: [w111] -> _
    shift-left: w1 -> [w116]
    shift-right: [w102] -> _
    shift-left: w1 -> [w115]
    shift-right: [w100] -> _
    shift-left: w1 -> [w114]
    shift-right: [w106] -> _
    shift-left: w1 -> [w113]
    shift-right: [w105] -> _
    shift-left: w1 -> [w112]
    shift-right: [w61] -> _
    shift-left: "Probe 4" -> [w192]
    shift-right: [w66] -> _
    shift-left: w1 -> [w91]
    shift-right: [w67] -> _
    shift-left: w1 -> [w90]
    shift-right: [w68] -> _
    shift-left: w1 -> [w89]
    shift-right: [w69] -> _
    shift-left: w1 -> [w88]
    i -> [w152]
    stop <- "Interrupt program" stop-if-true
    # "Ig for bias stress plots"
    # "Id for bias stress plots"
    # "Is for bias stress plots"
    # "Time axis for bias stress plots"
    # "Save bias stress curves in file."
    # "Is off"
    # "Is on"
    # "Ig off"
    # "Ig on"
    # "Is min"
    # "Is max"
    # "Ig min"
    # "Ig max"
    # "Id min"
    # "Id max"
    # "Id off"
    # "Id on"
    # "Is off"
    # "Is on"
    # "Ig off"
    # "Ig on"
    # "Is min"
    # "Is max"
    # "Ig min"
    # "Ig max"
    # "Id min"
    # "Id max"
    # "Id off"
    # "Id on"
    # "Filepath and name"
    # "Limit of command arguments (array columns). Raise if needed."
    # "Serial port data (string)"
    # "Serial port data (table)"
    # "Serial port data"
    # "For loop counter"
    # "<-----Equivalent to the 4155C \"Write\" subvi.----->"
    # "Headers"
    # "Save transfer curves in file."
    # "Filepath and name"
    # "Save time-dependent data."
    # "Use the time offset if your measurements do not start at t=0."
    # "Time for Imax, Imin, Ion, Ioff"
    # "Rest of elements of command"
    # "First element of command\n(case select)"
    n20 = Add(x=w152, y=1) -> (x+y=→"Line running":i32)
    n21 = Add(x=w157, y=1) -> (x+y=→"Total lines":i32)
    n22 = Index Array(array=w185, index=0 ("line index")) -> (element=w180:string)
    "Command running:" <- w180
    n23 = control-ref of="Interrupt scan"() -> (w204:refnum<vi>)
    n24 = Spreadsheet String To Array(delimiter (Tab)=" ", format string="%s", spreadsheet string=w180, array type (2D Dbl)=string[] []) -> (array=w178:string[])
    n25 = Delete From Array(array=w178, index=0) -> (deleted portion=w132:string, array with subset deleted=w177:string[])  [unwired: 1 in]
    n26 = call "Elapsed Time"("Reset"="Reset", "Auto Reset"="Auto Reset") -> ("Elapsed Time (s)"=w187:dbl)  [unwired: 10 in, 7 out]
    n27 = case shown="2" "Time Units" {
      tunnel: ["-sec" "-min" "-h"] -> w188
      tunnel: [w217 w221 w224] -> w158
      tunnel: w187 -> [w217 w220 w225]
      frame 0, Default {
      }
      frame 1 {
        n28 = Divide(x=w220, y=60.0) -> (x/y=w221:dbl)
      }
      frame 2 {
        n29 = Divide(x=w225, y=3600.0) -> (x/y=w224:dbl)
      }
    }
    n30 = Add(x=w158, y="Time Offset") -> (x+y=w92:dbl)
    n31 = To Long Integer(number=w92) -> (32bit integer=w93:i32)
    "Elapsed Time" <- w93
    n32 = case shown="\"sample\"" w132 {
      tunnel: w177 -> [w261 w298 w334 w350 w476 w593 w737 w861 w1026 w1058 w1131 w1176 w1219 w1258 w1290 _ _ w1476 w1608 _ w1712 w1776 w1837 w1930 w2010 w2048]
      tunnel: w213 -> [w256 w294 w332 w363 w483 w652 w745 w868 w1034 w1075 w1120 w1168 w1212 w1252 w1283 w1320 w1380 w1457 w1590 w1639 w1699 w1763 w1825 w1924 w2006 w2050]
      tunnel: w212 -> [w255 w293 w323 w362 w454 w637 w714 w839 w1002 w1076 w1121 w1169 w1213 w1253 w1284 w1325 w1382 w1482 w1614 w1643 w1718 w1782 w1843 w1936 w1964 w2054]
      tunnel: w211 -> [w254 w292 w322 w361 w453 w636 w713 w838 w999 w1077 w1122 w1170 w1214 w1254 w1285 w1324 w1353 w1481 w1613 w1642 w1717 w1781 w1842 w1935 w1963 w2053]
      tunnel: w210 -> [w253 w291 w331 w359 w479 w613 w741 w864 w1030 w1085 w1130 w1167 w1211 w1251 w1282 w1323 w1377 w1449 w1582 w1648 w1692 w1756 w1818 w1923 w2005 w2055]
      tunnel: w209 -> [w252 w290 w330 w358 w481 w650 w743 w866 w1032 w1084 w1129 w1175 w1218 w1257 w1289 w1322 w1362 w1480 w1612 w1651 w1716 w1780 w1841 w1934 w2014 w2056]
      tunnel: w208 -> [w251 w289 w329 w356 w480 w649 w742 w865 w1031 w1083 w1128 w1174 w1217 w1256 w1288 w1321 w1363 w1458 w1591 w1650 w1700 w1764 w1826 w1925 w2007 w2058]
      tunnel: [w255 w293 w321 w362 w478 w647 w739 w863 w1028 w1076 w1121 w1169 w1213 w1253 w1284 w1325 w1382 w1450 w1564 w1641 w1693 w1757 w1819 w1877 w1966 w2054] -> w207
      tunnel: [w254 w292 w320 w361 w477 w646 w738 w862 w1027 w1077 w1122 w1170 w1214 w1254 w1285 w1324 w1352 w1459 w1565 w1640 w1701 w1765 w1827 w1876 w1965 w2052] -> w143
      tunnel: [w253 w291 w331 w359 w479 w609 w741 w864 w1030 w1078 w1123 w1167 w1211 w1251 w1282 w1323 w1377 w1449 w1582 w1648 w1692 w1756 w1818 w1923 w2005 w2055] -> w62
      tunnel: [w252 w290 w330 w358 w481 w650 w743 w866 w1032 w1084 w1129 w1175 w1218 w1257 w1289 w1322 w1362 w1480 w1612 w1651 w1716 w1780 w1841 w1934 w2014 w2056] -> w206
      tunnel: [w251 w289 w329 w356 w480 w649 w742 w865 w1031 w1083 w1128 w1174 w1217 w1256 w1288 w1321 w1363 w1458 w1591 w1650 w1700 w1764 w1826 w1925 w2007 w2058] -> w205
      tunnel: [w256 w294 w332 w363 w483 w652 w745 w868 w1034 w1075 w1120 w1168 w1212 w1252 w1283 w1320 w1380 w1457 w1590 w1639 w1699 w1763 w1825 w1924 w2006 w2050] -> w70
      tunnel: w204 -> [_ _ _ _ w485 w656 w750 w870 w1038 _ _ _ _ _ _ _ _ w1454 w1587 _ w1698 w1762 w1824 w1896 w1982 _]
      tunnel: "Gate" -> [_ _ _ _ w463 w640 w724 w848 w1013 _ _ _ _ _ _ _ _ _ _ _ _ _ _ _ _ _]
      tunnel: "Drain 2" -> [_ _ _ _ w462 w639 w723 w847 w1012 _ _ _ _ _ _ _ _ _ _ _ _ _ _ _ _ _]
      tunnel: "Panel Controls" -> [_ _ _ _ _ _ w722 w774 w1011 _ _ _ _ _ _ _ _ _ _ _ _ _ _ _ _ _]
      tunnel: w200 -> [w250 w288 w328 w355 w447 w630 w707 w832 w997 w1082 w1127 _ w1210 w1250 w1281 w1319 w1364 w1445 w1578 w1644 w1688 w1752 w1814 w1919 w2001 w2059]
      tunnel: w199 -> [w249 w287 w327 w354 w446 w629 w706 w831 w996 w1081 w1126 w1173 _ w1241 w1287 w1318 w1365 w1446 w1579 w1645 w1689 w1753 w1815 w1920 w2002 w2060]
      tunnel: w198 -> [w248 w286 w326 w353 w445 w628 w705 w830 w995 w1080 w1125 w1172 w1216 w1255 _ w1317 w1366 w1447 w1580 w1646 w1690 w1754 w1816 w1921 w2003 w2061]
      tunnel: w197 -> [w247 w285 w325 w352 w444 w627 w704 w829 w998 w1079 w1124 w1171 w1215 _ w1286 w1316 w1367 w1448 w1581 w1647 w1691 w1755 w1817 w1922 w2004 w2062]
      tunnel: [w250 w288 w328 w355 w447 w630 w707 w832 w997 w1082 w1127 w1166 w1210 w1250 w1281 w1319 w1364 w1445 w1578 w1644 w1688 w1752 w1814 w1919 w2001 w2059] -> w196
      tunnel: [w249 w287 w327 w354 w446 w629 w706 w831 w996 w1081 w1126 w1173 w1202 w1241 w1287 w1318 w1365 w1446 w1579 w1645 w1689 w1753 w1815 w1920 w2002 w2060] -> w195
      tunnel: [w248 w286 w326 w353 w445 w628 w705 w830 w995 w1080 w1125 w1172 w1216 w1255 w1280 w1317 w1366 w1447 w1580 w1646 w1690 w1754 w1816 w1921 w2003 w2061] -> w194
      tunnel: [w247 w285 w325 w352 w444 w627 w704 w829 w998 w1079 w1124 w1171 w1215 w1242 w1286 w1316 w1367 w1448 w1581 w1647 w1691 w1755 w1817 w1922 w2004 w2062] -> w193
      tunnel: w192 -> [w231 w266 w303 _ w385 w582 w676 w770 w966 w1055 w1103 w1150 w1186 w1225 w1264 w1300 w1330 w1432 w1544 w1623 w1659 w1727 w1790 w1856 w1941 w2019]
      tunnel: w191 -> [_ _ _ _ w438 w624 _ _ _ _ _ _ _ _ _ _ _ _ _ _ _ _ _ _ _ _]
      tunnel: [w246 w281 w318 w367 w400 w601 w694 w786 w984 w1074 w1118 w1165 w1201 w1240 w1279 w1315 w1348 w1422 w1548 w1638 w1677 w1745 w1808 w1874 w1959 w2051] -> w110
      tunnel: w190 -> [w246 w281 w318 w367 w435 w601 w694 w821 w984 w1074 w1118 w1165 w1201 w1240 w1279 w1315 w1348 w1428 w1548 w1638 w1677 w1745 w1808 w1874 w1959 w2051]
      tunnel: w92 -> [_ _ _ _ w434 w598 w692 w820 w981 _ _ _ _ _ _ _ w1346 w1437 w1560 _ w1674 w1742 w1805 w1871 w1955 _]
      tunnel: w188 -> [_ _ _ _ w431 w597 w690 w817 w980 _ _ _ _ _ _ _ w1344 w1435 w1559 _ w1673 w1741 w1804 w1870 w1956 _]
      tunnel: w93 -> [_ _ _ _ w427 _ _ w813 _ _ _ _ _ _ _ _ _ _ _ _ _ _ _ _ _ _]
      tunnel: [w245 w280 w317 w357 w404 w600 w693 w790 w983 w1073 w1117 w1164 w1200 w1239 w1278 w1314 w1347 w1407 w1562 w1637 w1676 w1744 w1807 w1873 w1958 w2057] -> w144
      tunnel: w186 -> [w245 w280 w317 w357 w430 w600 w693 w816 w983 w1073 w1117 w1164 w1200 w1239 w1278 w1314 w1347 w1409 w1562 w1637 w1676 w1744 w1807 w1873 w1958 w2057]
      tunnel: [w244 w279 w316 w366 w399 w596 w689 w785 w979 w1072 w1116 w1163 w1199 w1238 w1277 w1313 w1343 w1421 w1547 w1636 w1672 w1740 w1803 w1869 w1954 w2046] -> w109
      tunnel: w162 -> [w244 w279 w316 w366 w426 w596 w689 w812 w979 w1072 w1116 w1163 w1199 w1238 w1277 w1313 w1343 w1427 w1547 w1636 w1672 w1740 w1803 w1869 w1954 w2046]
      tunnel: [w243 w278 w315 w351 w419 w595 w688 w805 w978 w1071 w1115 w1162 w1198 w1237 w1276 w1312 w1342 w1434 w1558 w1635 w1671 w1739 w1802 w1868 w1953 w2045] -> w139
      tunnel: w149 -> [w243 w278 w315 w351 w419 w595 w688 w805 w978 w1071 w1115 w1162 w1198 w1237 w1276 w1312 w1342 w1434 w1558 w1635 w1671 w1739 w1802 w1868 w1953 w2044]
      tunnel: [w242 w277 w314 w360 w418 w594 w687 w804 w977 w1070 w1114 w1161 w1197 w1236 w1275 w1311 w1341 w1433 w1557 w1634 w1670 w1738 w1801 w1867 w1952 w2030] -> w140
      tunnel: w142 -> [w242 w277 w314 w360 w418 w594 w687 w804 w977 w1070 w1114 w1161 w1197 w1236 w1275 w1311 w1341 w1433 w1557 w1634 w1670 w1738 w1801 w1867 w1952 w2030]
      tunnel: [w240 w275 w312 w372 w393 w591 w685 w779 w975 w1068 w1113 w1160 w1195 w1234 w1273 w1309 w1339 w1415 w1556 w1633 w1669 w1737 w1799 w1866 w1951 w2029] -> w103
      tunnel: w131 -> [w240 w275 w312 w372 w417 w591 w685 w803 w975 w1068 w1113 w1160 w1195 w1234 w1273 w1309 w1339 w1415 w1556 w1633 w1669 w1737 w1799 w1866 w1951 w2029]
      tunnel: [w241 w276 w313 w373 w394 w592 w686 w780 w976 w1069 w1112 w1159 w1196 w1235 w1274 w1310 w1340 w1416 w1555 w1632 w1668 w1736 w1800 w1865 w1950 w2028] -> w104
      tunnel: w130 -> [w241 w276 w313 w373 w416 w592 w686 w802 w976 w1069 w1112 w1159 w1196 w1235 w1274 w1310 w1340 w1416 w1555 w1632 w1668 w1736 w1800 w1865 w1950 w2028]
      tunnel: [w233 w268 w305 w365 w398 w588 w683 w784 w973 w1061 w1110 w1157 w1193 w1232 w1271 w1307 w1332 w1420 w1546 w1631 w1661 w1729 w1792 w1858 w1945 w2021] -> w108
      tunnel: w119 -> [w233 w268 w305 w365 w412 w588 w683 w798 w973 w1061 w1110 w1157 w1193 w1232 w1271 w1307 w1332 w1426 w1546 w1631 w1661 w1729 w1792 w1858 w1945 w2021]
      tunnel: [w232 w267 w304 w364 w397 w589 w684 w783 w974 w1060 w1111 w1158 w1194 w1233 w1272 w1308 w1331 w1419 w1545 w1630 w1660 w1728 w1791 w1857 w1944 w2020] -> w107
      tunnel: w118 -> [w232 w267 w304 w364 w411 w589 w684 w797 w974 w1060 w1111 w1158 w1194 w1233 w1272 w1308 w1331 w1425 w1545 w1630 w1660 w1728 w1791 w1857 w1944 w2020]
      tunnel: [w235 w270 w307 w369 w403 w587 w681 w789 w971 w1066 w1108 w1155 w1191 w1230 w1269 w1305 w1334 w1424 w1550 w1625 w1663 w1731 w1794 w1860 w1943 w2025] -> w101
      tunnel: w117 -> [w235 w270 w307 w369 w410 w587 w681 w796 w971 w1066 w1108 w1155 w1191 w1230 w1269 w1305 w1334 w1430 w1550 w1625 w1663 w1731 w1794 w1860 w1943 w2025]
      tunnel: [w234 w269 w306 w368 w401 w590 w682 w787 w972 w1067 w1109 w1156 w1192 w1231 w1270 w1306 w1333 w1423 w1549 w1624 w1662 w1730 w1793 w1859 w1942 w2024] -> w111
      tunnel: w116 -> [w234 w269 w306 w368 w409 w590 w682 w795 w972 w1067 w1109 w1156 w1192 w1231 w1270 w1306 w1333 w1429 w1549 w1624 w1662 w1730 w1793 w1859 w1942 w2024]
      tunnel: [w237 w272 w309 w371 w392 w586 w679 w778 w969 w1064 w1106 w1153 w1189 w1228 w1267 w1303 w1336 w1414 w1552 w1627 w1665 w1733 w1796 w1862 w1947 w2027] -> w102
      tunnel: w115 -> [w237 w272 w309 w371 w408 w586 w679 w794 w969 w1064 w1106 w1153 w1189 w1228 w1267 w1303 w1336 w1414 w1552 w1627 w1665 w1733 w1796 w1862 w1947 w2027]
      tunnel: [w236 w271 w308 w370 w391 w585 w680 w777 w970 w1065 w1107 w1154 w1190 w1229 w1268 w1304 w1335 w1413 w1551 w1626 w1664 w1732 w1795 w1861 w1946 w2026] -> w100
      tunnel: w114 -> [w236 w271 w308 w370 w407 w585 w680 w793 w970 w1065 w1107 w1154 w1190 w1229 w1268 w1304 w1335 w1413 w1551 w1626 w1664 w1732 w1795 w1861 w1946 w2026]
      tunnel: [w239 w274 w311 w375 w396 w584 w677 w782 w967 w1062 w1104 w1151 w1187 w1226 w1265 w1301 w1338 w1418 w1554 w1629 w1667 w1735 w1798 w1864 w1949 w2023] -> w106
      tunnel: w113 -> [w239 w274 w311 w375 w406 w584 w677 w792 w967 w1062 w1104 w1151 w1187 w1226 w1265 w1301 w1338 w1418 w1554 w1629 w1667 w1735 w1798 w1864 w1949 w2023]
      tunnel: [w238 w273 w310 w374 w395 w583 w678 w781 w968 w1063 w1105 w1152 w1188 w1227 w1266 w1302 w1337 w1417 w1553 w1628 w1666 w1734 w1797 w1863 w1948 w2022] -> w105
      tunnel: w112 -> [w238 w273 w310 w374 w405 w583 w678 w791 w968 w1063 w1105 w1152 w1188 w1227 w1266 w1302 w1337 w1417 w1553 w1628 w1666 w1734 w1797 w1863 w1948 w2022]
      tunnel: [w231 w266 w303 w341 w385 w582 w676 w770 w966 w1055 w1103 w1150 w1186 w1225 w1264 w1300 w1330 w1432 w1544 w1623 w1659 w1727 w1790 w1856 w1941 w2019] -> w61
      tunnel: w92 -> [_ _ _ _ _ _ _ _ _ _ _ _ _ _ _ _ _ w1384 _ _ _ _ _ _ _ _]
      tunnel: [w230 w265 w302 w340 w384 w581 w675 w769 w965 w1054 w1102 w1149 w1185 w1224 w1263 w1299 w1329 w1396 w1543 w1622 w1658 w1726 w1789 w1855 w1940 w2018] -> w66
      tunnel: [w229 w264 w301 w339 w383 w580 w674 w768 w964 w1053 w1101 w1148 w1184 w1223 w1262 w1298 w1328 w1393 w1542 w1621 w1657 w1725 w1788 w1854 w1939 w2017] -> w67
      tunnel: [w228 w263 w300 w338 w382 w579 w673 w767 w963 w1052 w1100 w1147 w1183 w1222 w1261 w1297 w1327 w1394 w1541 w1620 w1656 w1724 w1787 w1853 w1938 w2016] -> w68
      tunnel: [w227 w262 w299 w337 w381 w578 w672 w766 w962 w1051 w1099 w1146 w1182 w1221 w1260 w1296 w1326 w1395 w1540 w1619 w1655 w1723 w1786 w1852 w1937 w2015] -> w69
      tunnel: w91 -> [w230 w265 w302 w340 w384 w581 w675 w769 w965 w1054 w1102 w1149 w1185 w1224 w1263 w1299 w1329 w1400 w1543 w1622 w1658 w1726 w1789 w1855 w1940 w2018]
      tunnel: w90 -> [w229 w264 w301 w339 w383 w580 w674 w768 w964 w1053 w1101 w1148 w1184 w1223 w1262 w1298 w1328 w1399 w1542 w1621 w1657 w1725 w1788 w1854 w1939 w2017]
      tunnel: w89 -> [w228 w263 w300 w338 w382 w579 w673 w767 w963 w1052 w1100 w1147 w1183 w1222 w1261 w1297 w1327 w1398 w1541 w1620 w1656 w1724 w1787 w1853 w1938 w2016]
      tunnel: w88 -> [w227 w262 w299 w337 w381 w578 w672 w766 w962 w1051 w1099 w1146 w1182 w1221 w1260 w1296 w1326 w1397 w1540 w1619 w1655 w1723 w1786 w1852 w1937 w2015]
      tunnel: "Standby" -> [_ _ _ _ w380 w577 _ w765 _ _ _ _ _ _ _ _ _ w1391 w1539 _ _ _ _ w1851 _ _]
      frame "wait" {
        n33 = Index Array(array=w261, index=0 ("Index")) -> (element=w259:string)
        n34 = Decimal String To Number(string=w259, default (0L)=u32 0) -> (number=w258:u32)  [unwired: 1 in, 1 out]
        n35 = Wait (ms)(milliseconds to wait=w258) -> ()  [unwired: 1 out]
      }
      frame "wait-min" {
        n36 = Index Array(array=w298, index=0 ("Index")) -> (element=w296:string)
        n37 = Decimal String To Number(string=w296, default (0L)=u32 0) -> (number=w284:u32)  [unwired: 1 in, 1 out]
        n38 = Multiply(x=w284, y=u32 60000) -> (x*y=w283:u32)
        n39 = Wait (ms)(milliseconds to wait=w283) -> ()  [unwired: 1 out]
      }
      frame "standby" {
        n40 = Index Array(array=w334, index=0 ("Index")) -> (element=w324:string)
        n41 = case shown="\"off\", Default" w324 {
          tunnel: [":PAGE:SCON:STAN 0" ":PAGE:SCON:STAN 1"] -> w319
          frame "off", Default {
          }
          frame "on" {
          }
        }
        n42 = VISA Write(VISA resource name=w323, write buffer=w319, error in (no error)=w322) -> (VISA resource name out=w321:refnum<visa-resource-name>, error out=w320:errorcluster)  [unwired: 1 out]
      }
      frame "Probe4" {
        n43 = Delete From Array(array=w350, index=0) -> (deleted portion=w344:string, array with subset deleted=w347:string[])  [unwired: 1 in]
        n44 = Equal?(x=w344, y="ON") -> (x = y?=w342:bool)
        n45 = Delete From Array(array=w347, index=0) -> (deleted portion=w346:string)  [unwired: 1 in, 1 out]
        n46 = Fract/Exp String To Number(string=w346) -> (number=w343:dbl)  [unwired: 3 in, 1 out]
        n47 = Bundle(w342, w343) -> (w341:cluster{bool, dbl})  [unwired: 1 in]
      }
      frame "transfer" {
        n48 = local read "Transfer/Output - Gate"() -> (w379:u32)
        n49 = Delete From Array(array=w476, index=0 ("Index")) -> (deleted portion=w474:string, array with subset deleted=w473:string[])  [unwired: 1 in]
        n50 = Bundle By Name(cluster=w438, "Emergency Stop"=w485) -> (w439:T2)
        n51 = Number To Decimal String(number=w434) -> (decimal integer string=w433:string)  [unwired: 1 in]
        n52 = case shown="\"d\", Default" w474 {
          tunnel: [w570 w571] -> w472
          frame "s" {
            w570 = u16 0 items=["Single", "Double"] ("sweep mode")
          }
          frame "d", Default {
            w571 = u16 1 items=["Single", "Double"] ("sweep mode")
          }
        }
        n53 = Fract/Exp String To Number(string=w473) -> (number=w458:dbl[])  [unwired: 3 in, 1 out]
        n54 = Concatenate Strings(w483, "-transfer-" ("Prefix"), w433, w431, ".txt" ("Suffix (transfer)")) -> (w484:string)
        n55 = VISA Write(VISA resource name=w454, write buffer=":PAGE:CHAN:MODE SWE;" ("write buffer (\"\")"), error in (no error)=w453) -> (VISA resource name out=w451:refnum<visa-resource-name>, error out=w452:errorcluster)  [unwired: 1 out]
        n56 = local read "Plot transfer curve extrema vs time"() -> (w386:bool)
        n57 = String To Path(string=w484) -> (path=w482:path)
        n58 = Index Array(array=w458, index #1=0 ("Index")) -> (element #1=w471:dbl, element #2=w470:dbl, element #3=w469:dbl)  [unwired: 2 in]
        n59 = Delete From Array(array=w458, length=3 ("Length"), index=0 ("Index")) -> (array with subset deleted=w456:dbl[])  [unwired: 1 out]
        n60 = local read "Transfer/Output - Drain"() -> (w376:u32)
        n61 = local read "Transfer/Output - Source/Common"() -> (w378:u32)
        n62 = case shown="True" w386 {
          tunnel: w430 -> [w487 w490]
          tunnel: w427 -> [_ w489]
          tunnel: [w487 w488] -> w404
          frame False {
          }
          frame True {
            n63 = Build Array (concatenate)(w490, w489) -> (w488:i32[])
          }
        }
        n64 = local read "Transfer/Output - Probe 4"() -> (w377:u32)
        n65 = Bundle By Name(cluster=w463, "Gate Start"=w471, "Gate Stop"=w470, "Gate Step (linear only)"=w469, "Gate Compliance"=w480, "Range mode"=w447, "Range"=w446) -> (w448:T6)
        n66 = Index Array(array=w456, index #1=0 ("Index")) -> (element #1=w466:dbl, element #2=w465:dbl, element #3=w464:dbl)  [unwired: 2 in]
        n67 = call <vilib>:"compatOverwrite.vi"("overwrite (F)"=TRUE) -> ("overwrite?"=w437:T8)
        n68 = Bundle By Name(cluster=w462, "Drain Start"=w466, "Drain Stop"=w465, "Drain Step"=w464, "Drain Compliance"=w481, "Range mode"=w445, "Range"=w444) -> (w449:T7)
        n69 = call "4155C Transfer v3.0.vi"("VISA resource name in"=w451, "Source/Common"=w378, 2:"Gate"=w448, 3:"Drain"=w449, 4:"Drain"=w376, "Timings"=w479, "error in (no error)"=w452, 7:"Probe 4"=w385, 8:"Gate"=w379, 9:"Probe 4"=w377, "sweep mode"=w472, "Panel Controls"=w439, "Standby"=w380) -> ("VG"=w436:dbl[], "Outparams"=w443:T9, "VISA Resource Name out"=w478:refnum<visa-resource-name>, "IS"=w414:dbl[], "ID"=w415:dbl[], "IG"=w413:dbl[], "error out"=w428:errorcluster, "Probe 4"=w440:dbl[])  [unwired: 7 in]
        n70 = Unbundle By Name(w443) -> ("V2 Step"=w442:dbl, "V2 Start"=w441:dbl, "Number of points"=w402:i32)
        n71 = call "4155C Split array.vi"("Number of VAR2 steps"=w402, "Y2 data in"=w415, "X data in"=w436, "Y1 data in"=w414, "Y3 data in"=w413, "error in (no error)"=w428) -> ("Array of clusters"=w429:cluster{"Y data in":dbl[], "X data in":dbl[]}[], "error out"=w390:errorcluster)  [unwired: 1 in]
        n72 = case shown="True" "Plot transfer curve extrema vs time" {
          tunnel: w435 -> [w493 w569]
          tunnel: w426 -> [w494 w564]
          tunnel: w417 -> [w500 w560]
          tunnel: w416 -> [w501 w559]
          tunnel: w415 -> [_ w556]
          tunnel: w414 -> [_ w554]
          tunnel: w413 -> [_ w553]
          tunnel: w412 -> [w495 w549]
          tunnel: w411 -> [w497 w548]
          tunnel: w410 -> [w491 w545]
          tunnel: w409 -> [w492 w544]
          tunnel: w408 -> [w499 w541]
          tunnel: w407 -> [w498 w540]
          tunnel: w406 -> [w503 w537]
          tunnel: w405 -> [w502 w536]
          tunnel: w404 -> [_ w529]
          tunnel: [w491 w524] -> w403
          tunnel: w402 -> [_ w523]
          tunnel: [w492 w522] -> w401
          tunnel: [w493 w521] -> w400
          tunnel: [w494 w520] -> w399
          tunnel: [w495 w519] -> w398
          tunnel: [w497 w518] -> w397
          tunnel: [w503 w517] -> w396
          tunnel: [w502 w516] -> w395
          tunnel: [w501 w515] -> w394
          tunnel: [w500 w514] -> w393
          tunnel: [w499 w513] -> w392
          tunnel: [w498 w512] -> w391
          tunnel: w390 -> [w496 w511]
          tunnel: [w496 w507] -> w389
          frame False {
          }
          frame True {
            # "Adjusts graph colors."
            # "Adjusts graph colors."
            # "Ion will be the middle element of the array. The calculation of the index is done only once, since Is, Id, and Ig have the same dimensions."
            # "abs(Ig)"
            # "abs(Is)"
            # "Y1: Is\nY2: Id\nY3: Ig"
            # "abs(Id)"
            # "Adjusts graph colors."
            # "Adjusts graph colors."
            # "Adjusts graph colors."
            n73 = Absolute Value(x=w554) -> (abs(x)=w539:dbl[])
            n74 = Absolute Value(x=w556) -> (abs(x)=w555:dbl[])
            n75 = Absolute Value(x=w553) -> (abs(x)=w542:dbl[])
            n76 = Array Size(array=w555) -> (size(s)=w563:i32)
            n77 = Divide(x=w563, y=2) -> (x/y=w506:dbl)
            n78 = Subtract(x=w506, y=1) -> (x-y=w505:dbl)
            n79 = Array Max & Min(array=w539) -> (max value=w546:dbl, min value=w547:dbl)  [unwired: 2 out]
            n80 = Array Max & Min(array=w555) -> (max value=w568:dbl, min value=w552:dbl)  [unwired: 2 out]
            n81 = Array Max & Min(array=w542) -> (max value=w551:dbl, min value=w550:dbl)  [unwired: 2 out]
            n82 = Index Array(array=w539, index=w505) -> (element=w530:dbl)
            n83 = Index Array(array=w539, index=0) -> (element=w531:dbl)
            n84 = Index Array(array=w555, index=w505) -> (element=w532:dbl)
            n85 = Index Array(array=w555, index=0) -> (element=w533:dbl)
            n86 = Index Array(array=w542, index=w505) -> (element=w535:dbl)
            n87 = Index Array(array=w542, index=0) -> (element=w534:dbl)
            n88 = local write "Ig max"(w551) -> ()
            n89 = local write "Ig min"(w550) -> ()
            n90 = local write "Is max"(w546) -> ()
            n91 = local write "Is min"(w547) -> ()
            n92 = local write "Id max"(w568) -> ()
            n93 = local write "Id min"(w552) -> ()
            n94 = Build Array (concatenate)(w545, w546) -> (w524:dbl[])
            n95 = Build Array (concatenate)(w544, w547) -> (w522:dbl[])
            n96 = local write "Is off"(w531) -> ()
            n97 = local write "Is on"(w530) -> ()
            n98 = Build Array (concatenate)(w569, w568) -> (w521:dbl[])
            n99 = Build Array (concatenate)(w564, w552) -> (w520:dbl[])
            n100 = Build Array (concatenate)(w549, w551) -> (w519:dbl[])
            n101 = Build Array (concatenate)(w548, w550) -> (w518:dbl[])
            n102 = Build Array (concatenate)(w537, w530) -> (w517:dbl[])
            n103 = Build Array (concatenate)(w536, w531) -> (w516:dbl[])
            n104 = Build Array (concatenate)(w559, w532) -> (w515:dbl[])
            n105 = Build Array (concatenate)(w560, w533) -> (w514:dbl[])
            n106 = Build Array (concatenate)(w541, w535) -> (w513:dbl[])
            n107 = Build Array (concatenate)(w540, w534) -> (w512:dbl[])
            n108 = local write "Ig off"(w534) -> ()
            n109 = local write "Ig on"(w535) -> ()
            n110 = local write "Id off"(w533) -> ()
            n111 = local write "Id on"(w532) -> ()
            n112 = control-ref of="Imax vs time"() -> (w558:refnum<vi>)
            n113 = control-ref of="Imin vs time"() -> (w557:refnum<vi>)
            n114 = control-ref of="Ion vs time"() -> (w526:refnum<vi>)
            n115 = control-ref of="Ioff vs time"() -> (w525:refnum<vi>)
            n116 = control-ref of="I vs Vg"() -> (w567:refnum<vi>)
            n117 = call "4155C Split array.vi"("Number of VAR2 steps"=w523, "Y2 data in"=w515, "X data in"=w529, "Y1 data in"=w517, "Y3 data in"=w513, "error in (no error)"=w511) -> ("Array of clusters"=w527:cluster{"Y data in":dbl[], "X data in":dbl[]}[], "error out"=w510:errorcluster)  [unwired: 1 in]
            n118 = call "4155C Split array.vi"("Number of VAR2 steps"=w523, "Y2 data in"=w514, "X data in"=w529, "Y1 data in"=w516, "Y3 data in"=w512, "error in (no error)"=w510) -> ("Array of clusters"=w528:cluster{"Y data in":dbl[], "X data in":dbl[]}[], "error out"=w509:errorcluster)  [unwired: 1 in]
            n119 = call "4155C Split array.vi"("Number of VAR2 steps"=w523, "Y2 data in"=w521, "X data in"=w529, "Y1 data in"=w524, "Y3 data in"=w519, "error in (no error)"=w509) -> ("Array of clusters"=w566:cluster{"Y data in":dbl[], "X data in":dbl[]}[], "error out"=w508:errorcluster)  [unwired: 1 in]
            n120 = call "4155C Split array.vi"("Number of VAR2 steps"=w523, "Y2 data in"=w520, "X data in"=w529, "Y1 data in"=w522, "Y3 data in"=w518, "error in (no error)"=w508) -> ("Array of clusters"=w565:cluster{"Y data in":dbl[], "X data in":dbl[]}[], "error out"=w507:errorcluster)  [unwired: 1 in]
            n121 = call "4155C Config Chart Colours.vi"("Numeric"=w523, "XY Graph 2"=w558) -> ()  [unwired: 6 in]
            n122 = call "4155C Config Chart Colours.vi"("Numeric"=w523, "XY Graph 2"=w557) -> ()  [unwired: 6 in]
            n123 = call "4155C Config Chart Colours.vi"("Numeric"=w523, "XY Graph 2"=w526) -> ()  [unwired: 6 in]
            n124 = call "4155C Config Chart Colours.vi"("Numeric"=w523, "XY Graph 2"=w525) -> ()  [unwired: 6 in]
            n125 = call "4155C Config Chart Colours.vi"("Numeric"=w523, "XY Graph 2"=w567) -> ()  [unwired: 6 in]
            n126 = local write "Imax vs time"(w566) -> ()
            n127 = local write "Imin vs time"(w565) -> ()
            n128 = local write "Ion vs time"(w527) -> ()
            n129 = local write "Ioff vs time"(w528) -> ()
          }
        }
        n130 = local write "I vs Vg"(w429) -> ()
        n131 = Open/Create/Replace File(file path (use dialog)=w482, error in=w389, operation (0:open)=w437) -> (refnum out=w424:refnum<file>, error out=w422:errorcluster)  [unwired: 3 in, 1 out]
        n132 = call "4155C Make Big 2d array.vi"("1D Var1"=w436, "1d IS"=w414, "1d ID"=w415, "1d IG"=w413, "1d SMU4"=w440, "SMU4"=w385, "VAR2 START"=w441, "Number of VAR2 steps"=w402, "VAR2 STEP"=w442, "VAR1 Name"="Vg", "Decimal places in header"=i8 1, "VAR2 Name"="Vd") -> ("Header array"=w425:string[], "Data array"=w423:dbl[][])  [unwired: 14 in]
        n133 = call "4155C Write array to file.vi"("Byte Stream File Refnum"=w424, "Header"=w425, "Data Array"=w423, "error in (no error)"=w422) -> ("dup refnum"=w421:refnum<file>, "error out"=w420:errorcluster)  [unwired: 1 in]
        n134 = Close File(refnum=w421, error in=w420) -> (error out=w477:errorcluster)  [unwired: 1 out]
      }
      frame "pulsedstressV" {
        w607 = 0
        n135 = local read "Pulsed Stress V - Vextra"() -> (w574:u32)
        n136 = local read "Pulsed Stress V - Drain"() -> (w576:u32)
        n137 = local read "Pulsed Stress V - Gate"() -> (w573:u32)
        n138 = local read "Pulsed Stress V - Probe 4"() -> (w575:u32)
        n139 = local read "Pulsed Stress V - Source/Common"() -> (w572:u32)
        n140 = Number To Decimal String(number=w598) -> (decimal integer string=w653:string)  [unwired: 1 in]
        n141 = Delete From Array(array=w593, index=0 ("Index")) -> (deleted portion=w644:string, array with subset deleted=w643:string[])  [unwired: 1 in]
        n142 = Bundle By Name(cluster=w624, "Emergency Stop"=w656) -> (w625:T2)
        n143 = VISA Write(VISA resource name=w637, write buffer=":PAGE:CHAN:MODE SWE;" ("write buffer (\"\")"), error in (no error)=w636) -> (VISA resource name out=w634:refnum<visa-resource-name>, error out=w635:errorcluster)  [unwired: 1 out]
        n144 = Concatenate Strings(w652, "-pulsedstressV-" ("Substring"), w653, w597, ".txt" ("Substring")) -> (w655:string)
        n145 = case shown="\"d\", Default" w644 {
          tunnel: [w665 w666] -> w642
          frame "s" {
            w665 = u16 0 items=["Single", "Double"] ("sweep mode")
          }
          frame "d", Default {
            w666 = u16 1 items=["Single", "Double"] ("sweep mode")
          }
        }
        n146 = Fract/Exp String To Number(string=w643) -> (number=w638:dbl[])  [unwired: 3 in, 1 out]
        n147 = String To Path(string=w655) -> (path=w651:path)
        n148 = Index Array(array=w638, index #1=0 ("Index")) -> (element #1=w616:dbl, element #2=w615:dbl, element #3=w612:dbl, element #4=w611:dbl, element #5=w610:dbl, element #6=w614:dbl)  [unwired: 5 in]
        n149 = Bundle By Name(cluster=w613, "Pulse period"=w611, "Base voltage"=w612, "Pulse width"=w610) -> (w609:T4)
        n150 = Unbundle By Name(w609) -> ("Pulse period"=w617:dbl)
        n151 = Bundle By Name(cluster=w640, "Gate Start"=w615, "Gate Stop"=w616, "Gate Step (linear only)"=0, "Gate Compliance"=w649, "Range mode"=w630, "Range"=w629) -> (w631:T6)
        n152 = call <vilib>:"compatOverwrite.vi"("overwrite (F)"=TRUE) -> ("overwrite?"=w602:T8)
        n153 = Bundle By Name(cluster=w639, "Drain Start"=w614, "Drain Stop"=w607, "Drain Step"=w607, "Drain Compliance"=w650, "Range mode"=w628, "Range"=w627) -> (w632:T7)
        n154 = call "4155C PulsedStressV v3.0.vi"("VISA resource name in"=w634, "Gate"=w631, "Pulsed Stress V - Source/Common"=w572, "Drain"=w632, "Timings"=w609, "error in (no error)"=w635, "sweep mode"=w642, "Probe 4"=w582, "Pulsed Stress V - Drain"=w576, "Pulsed Stress V - Gate"=w573, "Panel Controls"=w625, "Standby"=w577, "Pulsed Stress V - Probe 4"=w575, "Pulsed Stress V - Vextra"=w574) -> ("Outparams"=w626:T9, "VISA Resource Name out"=w647:refnum<visa-resource-name>, "ID"=w605:dbl[], "IG"=w603:dbl[], "error out"=w648:errorcluster)  [unwired: 1 in]
        n155 = Unbundle By Name(w626) -> ("Number of points"=w604:i32)  [unwired: 2 out]
        n156 = for {
          N: w604 -> [_]
          tunnel: [w662] -> w606 mode=indexing
          tunnel: w617 -> [w664]
          i -> [w663]
          n157 = Multiply(x=w664, y=w663) -> (x*y=w662:dbl)
        }
        n158 = Insert Into Array(array=dbl[][] [] ("Input Array"), new element=w606) -> (w618:dbl[][])  [unwired: 2 in]
        n159 = Insert Into Array(array=w618, new element=w605) -> (w623:dbl[][])  [unwired: 2 in]
        n160 = Insert Into Array(array=w623, new element=w603) -> (w622:dbl[][])  [unwired: 2 in]
        n161 = Transpose 2D Array(2D array=w622) -> (transposed array=w621:dbl[][])
        n162 = Open/Create/Replace File(file path (use dialog)=w651, error in=w648, operation (0:open)=w602) -> (refnum out=w659:refnum<file>, error out=w660:errorcluster)  [unwired: 3 in, 1 out]
        n163 = call "4155C Write array to file.vi"("Byte Stream File Refnum"=w659, "Header"=string[] ["Time /s", "Id /A", "Ig /A"], "Data Array"=w621, "error in (no error)"=w660) -> ("dup refnum"=w657:refnum<file>, "error out"=w658:errorcluster)  [unwired: 1 in]
        n164 = Close File(refnum=w657, error in=w658) -> (error out=w646:errorcluster)  [unwired: 1 out]
      }
      frame "transfer-fpp" {
        n165 = local read "FPP - Source"() -> (w671:u32)
        n166 = local read "FPP - Drain"() -> (w669:u32)
        n167 = local read "FPP - Gate"() -> (w670:u32)
        n168 = local read "FPP - Probe 1"() -> (w667:u32)
        n169 = local read "FPP - Probe 2"() -> (w668:u32)
        n170 = Number To Decimal String(number=w692) -> (decimal integer string=w746:string)  [unwired: 1 in]
        n171 = Bundle By Name(cluster=w722, "Emergency Stop"=w750) -> (w758:T1)
        n172 = Delete From Array(array=w737, index=0 ("Index")) -> (deleted portion=w735:string, array with subset deleted=w734:string[])  [unwired: 1 in]
        n173 = Concatenate Strings(w745, "-transferfpp-" ("Substring"), w746, w690, ".txt" ("Substring")) -> (w748:string)
        n174 = VISA Write(VISA resource name=w714, write buffer=":PAGE:CHAN:MODE SWE;" ("write buffer (\"\")"), error in (no error)=w713) -> (VISA resource name out=w711:refnum<visa-resource-name>, error out=w712:errorcluster)  [unwired: 1 out]
        n175 = case shown="\"d\", Default" w735 {
          tunnel: [w759 w760] -> w733
          frame "s" {
            w759 = u16 0 items=["Single", "Double"] ("sweep mode")
          }
          frame "d", Default {
            w760 = u16 1 items=["Single", "Double"] ("sweep mode")
          }
        }
        n176 = Fract/Exp String To Number(string=w734) -> (number=w718:dbl[])  [unwired: 3 in, 1 out]
        n177 = String To Path(string=w748) -> (path=w744:path)
        n178 = Index Array(array=w718, index #1=0 ("Index")) -> (element #1=w732:dbl, element #2=w731:dbl, element #3=w730:dbl)  [unwired: 2 in]
        n179 = Delete From Array(array=w718, length=3 ("Length"), index=0 ("Index")) -> (array with subset deleted=w716:dbl[])  [unwired: 1 out]
        n180 = Bundle By Name(cluster=w724, "Gate Start"=w732, "Gate Stop"=w731, "Gate Step (linear only)"=w730, "Gate Compliance"=w742, "Range mode"=w707, "Range"=w706) -> (w708:T6)
        n181 = Index Array(array=w716, index #1=0 ("Index")) -> (element #1=w727:dbl, element #2=w726:dbl, element #3=w725:dbl)  [unwired: 2 in]
        n182 = call <vilib>:"compatOverwrite.vi"("overwrite (F)"=TRUE) -> ("overwrite?"=w695:T8)
        n183 = Bundle By Name(cluster=w723, "Drain Start"=w727, "Drain Stop"=w726, "Drain Step"=w725, "Drain Compliance"=w743, "Range mode"=w705, "Range"=w704) -> (w709:T7)
        n184 = call "4155C Transfer-FPP v3.0.vi"("VISA resource name in"=w711, "FPP - Source"=w671, "Gate"=w708, "Drain"=w709, "FPP - Drain"=w669, "Timings"=w741, "error in (no error)"=w712, "FPP - Gate"=w670, "FPP - Probe 1"=w667, "sweep mode"=w733, "FPP - Probe 2"=w668, "Panel Controls"=w758) -> ("VG"=w749:dbl[], "Outparams"=w703:T9, "VISA Resource Name out"=w739:refnum<visa-resource-name>, "Vprobe2"=w699:dbl[], "ID"=w698:dbl[], "IG"=w697:dbl[], "Vprobe1"=w696:dbl[], "error out"=w740:errorcluster)  [unwired: 8 in]
        n185 = Unbundle By Name(w703) -> ("V2 Step"=w702:dbl, "V2 Start"=w701:dbl, "Number of points"=w700:i32)
        n186 = Open/Create/Replace File(file path (use dialog)=w744, error in=w740, operation (0:open)=w695) -> (refnum out=w755:refnum<file>, error out=w756:errorcluster)  [unwired: 3 in, 1 out]
        n187 = call "4155C Make Big 2d array FPP.vi"("1D Var1"=w749, "1d ID"=w698, "1d Vp2"=w699, "1d IG"=w697, "1d Vp1"=w696, "VAR2 START"=w701, "Number of VAR2 steps"=w700, "VAR2 STEP"=w702, "VAR1 Name"="Vg", "Decimal places in header"=i8 1, "VAR2 Name"="Vd") -> ("Header array"=w751:string[], "Data array"=w752:dbl[][])  [unwired: 15 in]
        n188 = call "4155C Write array to file.vi"("Byte Stream File Refnum"=w755, "Header"=w751, "Data Array"=w752, "error in (no error)"=w756) -> ("dup refnum"=w753:refnum<file>, "error out"=w754:errorcluster)  [unwired: 1 in]
        n189 = Close File(refnum=w753, error in=w754) -> (error out=w738:errorcluster)  [unwired: 1 out]
      }
      frame "output" {
        n190 = local read "Transfer/Output - Drain"() -> (w762:u32)
        n191 = local read "Transfer/Output - Source/Common"() -> (w761:u32)
        n192 = local read "Transfer/Output - Gate"() -> (w763:u32)
        n193 = Delete From Array(array=w861, index=0 ("Index")) -> (deleted portion=w859:string, array with subset deleted=w858:string[])  [unwired: 1 in]
        n194 = Bundle By Name(cluster=w774, "Emergency Stop"=w870) -> (w824:T1)
        n195 = Number To Decimal String(number=w820) -> (decimal integer string=w819:string)  [unwired: 1 in]
        n196 = case shown="\"d\", Default" w859 {
          tunnel: [w955 w956] -> w857
          frame "s" {
            w955 = u16 0 items=["Single", "Double"] ("sweep mode")
          }
          frame "d", Default {
            w956 = u16 1 items=["Single", "Double"] ("sweep mode")
          }
        }
        n197 = Fract/Exp String To Number(string=w858) -> (number=w843:dbl[])  [unwired: 3 in, 1 out]
        n198 = Concatenate Strings(w868, "-output-" ("Substring"), w819, w817, ".txt" ("Suffix (transfer)")) -> (w869:string)
        n199 = VISA Write(VISA resource name=w839, write buffer=":PAGE:CHAN:MODE SWE;" ("write buffer (\"\")"), error in (no error)=w838) -> (VISA resource name out=w836:refnum<visa-resource-name>, error out=w837:errorcluster)  [unwired: 1 out]
        n200 = String To Path(string=w869) -> (path=w867:path)
        n201 = Index Array(array=w843, index #1=0 ("Index")) -> (element #1=w856:dbl, element #2=w855:dbl, element #3=w854:dbl)  [unwired: 2 in]
        n202 = Delete From Array(array=w843, length=3 ("Length"), index=0 ("Index")) -> (array with subset deleted=w841:dbl[])  [unwired: 1 out]
        n203 = local read "Plot output curve extrema vs time"() -> (w771:bool)
        n204 = local read "Transfer/Output - Probe 4"() -> (w764:u32)
        n205 = Bundle By Name(cluster=w848, "Gate Start"=w856, "Gate Stop"=w855, "Gate Step (linear only)"=w854, "Gate Compliance"=w865, "Range mode"=w832, "Range"=w831) -> (w833:T6)
        n206 = case shown="True" w771 {
          tunnel: w816 -> [w872 w875]
          tunnel: w813 -> [_ w874]
          tunnel: [w872 w873] -> w790
          frame False {
          }
          frame True {
            n207 = Build Array (concatenate)(w875, w874) -> (w873:i32[])
          }
        }
        n208 = Index Array(array=w841, index #1=0 ("Index")) -> (element #1=w851:dbl, element #2=w850:dbl, element #3=w849:dbl)  [unwired: 2 in]
        n209 = call <vilib>:"compatOverwrite.vi"("overwrite (F)"=TRUE) -> ("overwrite?"=w823:T8)
        n210 = Bundle By Name(cluster=w847, "Drain Start"=w851, "Drain Stop"=w850, "Drain Step"=w849, "Drain Compliance"=w866, "Range mode"=w830, "Range"=w829) -> (w834:T7)
        n211 = call "4155C Output v3.0.vi"("VISA resource name in"=w836, "Source/Common"=w761, 2:"Gate"=w833, 3:"Drain"=w834, 4:"Drain"=w762, "Timings"=w864, "error in (no error)"=w837, 7:"Probe 4"=w770, 8:"Gate"=w763, 9:"Probe 4"=w764, "sweep mode"=w857, "Panel controls"=w824, "Standby"=w765) -> ("VD"=w822:dbl[], "Outparams"=w828:T9, "VISA Resource Name out"=w863:refnum<visa-resource-name>, "IS"=w800:dbl[], "ID"=w801:dbl[], "IG"=w799:dbl[], "error out"=w814:errorcluster, "Probe 4"=w825:dbl[])  [unwired: 7 in]
        n212 = Unbundle By Name(w828) -> ("V2 Step"=w827:dbl, "V2 Start"=w826:dbl, "Number of points"=w788:i32)
        n213 = call "4155C Split array.vi"("Number of VAR2 steps"=w788, "Y2 data in"=w801, "X data in"=w822, "Y1 data in"=w800, "Y3 data in"=w799, "error in (no error)"=w814) -> ("Array of clusters"=w815:cluster{"Y data in":dbl[], "X data in":dbl[]}[], "error out"=w776:errorcluster)  [unwired: 1 in]
        n214 = case shown="True" "Plot output curve extrema vs time" {
          tunnel: w821 -> [w884 w954]
          tunnel: w812 -> [w885 w949]
          tunnel: w803 -> [w879 w945]
          tunnel: w802 -> [w878 w944]
          tunnel: w801 -> [_ w941]
          tunnel: w800 -> [_ w939]
          tunnel: w799 -> [_ w938]
          tunnel: w798 -> [w886 w934]
          tunnel: w797 -> [w887 w933]
          tunnel: w796 -> [w882 w930]
          tunnel: w795 -> [w883 w929]
          tunnel: w794 -> [w880 w926]
          tunnel: w793 -> [w881 w925]
          tunnel: w792 -> [w876 w922]
          tunnel: w791 -> [w877 w921]
          tunnel: w790 -> [_ w914]
          tunnel: [w882 w909] -> w789
          tunnel: w788 -> [_ w908]
          tunnel: [w883 w907] -> w787
          tunnel: [w884 w906] -> w786
          tunnel: [w885 w905] -> w785
          tunnel: [w886 w904] -> w784
          tunnel: [w887 w903] -> w783
          tunnel: [w876 w902] -> w782
          tunnel: [w877 w901] -> w781
          tunnel: [w878 w900] -> w780
          tunnel: [w879 w899] -> w779
          tunnel: [w880 w898] -> w778
          tunnel: [w881 w897] -> w777
          tunnel: w776 -> [w888 w896]
          tunnel: [w888 w892] -> w775
          frame False {
          }
          frame True {
            # "Adjusts graph colors."
            # "Adjusts graph colors."
            # "Ion will be the middle element of the array. The calculation of the index is done only once, since Is, Id, and Ig have the same dimensions."
            # "abs(Ig)"
            # "abs(Is)"
            # "Y1: Is\nY2: Id\nY3: Ig"
            # "abs(Id)"
            # "Adjusts graph colors."
            # "Adjusts graph colors."
            # "Adjusts graph colors."
            n215 = Absolute Value(x=w939) -> (abs(x)=w924:dbl[])
            n216 = Absolute Value(x=w941) -> (abs(x)=w940:dbl[])
            n217 = Absolute Value(x=w938) -> (abs(x)=w927:dbl[])
            n218 = Array Size(array=w940) -> (size(s)=w948:i32)
            n219 = Divide(x=w948, y=2) -> (x/y=w891:dbl)
            n220 = Subtract(x=w891, y=1) -> (x-y=w890:dbl)
            n221 = Array Max & Min(array=w924) -> (max value=w931:dbl, min value=w932:dbl)  [unwired: 2 out]
            n222 = Array Max & Min(array=w940) -> (max value=w953:dbl, min value=w937:dbl)  [unwired: 2 out]
            n223 = Array Max & Min(array=w927) -> (max value=w936:dbl, min value=w935:dbl)  [unwired: 2 out]
            n224 = Index Array(array=w924, index=w890) -> (element=w915:dbl)
            n225 = Index Array(array=w924, index=0) -> (element=w916:dbl)
            n226 = Index Array(array=w940, index=w890) -> (element=w917:dbl)
            n227 = Index Array(array=w940, index=0) -> (element=w918:dbl)
            n228 = Index Array(array=w927, index=w890) -> (element=w920:dbl)
            n229 = Index Array(array=w927, index=0) -> (element=w919:dbl)
            n230 = local write "Ig max"(w936) -> ()
            n231 = local write "Ig min"(w935) -> ()
            n232 = local write "Is max"(w931) -> ()
            n233 = local write "Is min"(w932) -> ()
            n234 = local write "Id max"(w953) -> ()
            n235 = local write "Id min"(w937) -> ()
            n236 = Build Array (concatenate)(w930, w931) -> (w909:dbl[])
            n237 = Build Array (concatenate)(w929, w932) -> (w907:dbl[])
            n238 = local write "Is off"(w916) -> ()
            n239 = local write "Is on"(w915) -> ()
            n240 = Build Array (concatenate)(w954, w953) -> (w906:dbl[])
            n241 = Build Array (concatenate)(w949, w937) -> (w905:dbl[])
            n242 = Build Array (concatenate)(w934, w936) -> (w904:dbl[])
            n243 = Build Array (concatenate)(w933, w935) -> (w903:dbl[])
            n244 = Build Array (concatenate)(w922, w915) -> (w902:dbl[])
            n245 = Build Array (concatenate)(w921, w916) -> (w901:dbl[])
            n246 = Build Array (concatenate)(w944, w917) -> (w900:dbl[])
            n247 = Build Array (concatenate)(w945, w918) -> (w899:dbl[])
            n248 = Build Array (concatenate)(w926, w920) -> (w898:dbl[])
            n249 = Build Array (concatenate)(w925, w919) -> (w897:dbl[])
            n250 = local write "Ig off"(w919) -> ()
            n251 = local write "Ig on"(w920) -> ()
            n252 = local write "Id off"(w918) -> ()
            n253 = local write "Id on"(w917) -> ()
            n254 = control-ref of="Imax vs time"() -> (w943:refnum<vi>)
            n255 = control-ref of="Imin vs time"() -> (w942:refnum<vi>)
            n256 = control-ref of="Ion vs time"() -> (w911:refnum<vi>)
            n257 = control-ref of="Ioff vs time"() -> (w910:refnum<vi>)
            n258 = control-ref of="I vs Vg"() -> (w952:refnum<vi>)
            n259 = call "4155C Split array.vi"("Number of VAR2 steps"=w908, "Y2 data in"=w900, "X data in"=w914, "Y1 data in"=w902, "Y3 data in"=w898, "error in (no error)"=w896) -> ("Array of clusters"=w912:cluster{"Y data in":dbl[], "X data in":dbl[]}[], "error out"=w895:errorcluster)  [unwired: 1 in]
            n260 = call "4155C Split array.vi"("Number of VAR2 steps"=w908, "Y2 data in"=w899, "X data in"=w914, "Y1 data in"=w901, "Y3 data in"=w897, "error in (no error)"=w895) -> ("Array of clusters"=w913:cluster{"Y data in":dbl[], "X data in":dbl[]}[], "error out"=w894:errorcluster)  [unwired: 1 in]
            n261 = call "4155C Split array.vi"("Number of VAR2 steps"=w908, "Y2 data in"=w906, "X data in"=w914, "Y1 data in"=w909, "Y3 data in"=w904, "error in (no error)"=w894) -> ("Array of clusters"=w951:cluster{"Y data in":dbl[], "X data in":dbl[]}[], "error out"=w893:errorcluster)  [unwired: 1 in]
            n262 = call "4155C Split array.vi"("Number of VAR2 steps"=w908, "Y2 data in"=w905, "X data in"=w914, "Y1 data in"=w907, "Y3 data in"=w903, "error in (no error)"=w893) -> ("Array of clusters"=w950:cluster{"Y data in":dbl[], "X data in":dbl[]}[], "error out"=w892:errorcluster)  [unwired: 1 in]
            n263 = call "4155C Config Chart Colours.vi"("Numeric"=w908, "XY Graph 2"=w943) -> ()  [unwired: 6 in]
            n264 = call "4155C Config Chart Colours.vi"("Numeric"=w908, "XY Graph 2"=w942) -> ()  [unwired: 6 in]
            n265 = call "4155C Config Chart Colours.vi"("Numeric"=w908, "XY Graph 2"=w911) -> ()  [unwired: 6 in]
            n266 = call "4155C Config Chart Colours.vi"("Numeric"=w908, "XY Graph 2"=w910) -> ()  [unwired: 6 in]
            n267 = call "4155C Config Chart Colours.vi"("Numeric"=w908, "XY Graph 2"=w952) -> ()  [unwired: 6 in]
            n268 = local write "Imax vs time"(w951) -> ()
            n269 = local write "Imin vs time"(w950) -> ()
            n270 = local write "Ion vs time"(w912) -> ()
            n271 = local write "Ioff vs time"(w913) -> ()
          }
        }
        n272 = local write "I vs Vd"(w815) -> ()
        n273 = Open/Create/Replace File(file path (use dialog)=w867, error in=w775, operation (0:open)=w823) -> (refnum out=w810:refnum<file>, error out=w808:errorcluster)  [unwired: 3 in, 1 out]
        n274 = call "4155C Make Big 2d array.vi"("1D Var1"=w822, "1d IS"=w800, "1d ID"=w801, "1d IG"=w799, "1d SMU4"=w825, "SMU4"=w770, "VAR2 START"=w826, "Number of VAR2 steps"=w788, "VAR2 STEP"=w827, "VAR1 Name"="Vd", "Decimal places in header"=i8 1, "VAR2 Name"="Vg") -> ("Header array"=w811:string[], "Data array"=w809:dbl[][])  [unwired: 14 in]
        n275 = call "4155C Write array to file.vi"("Byte Stream File Refnum"=w810, "Header"=w811, "Data Array"=w809, "error in (no error)"=w808) -> ("dup refnum"=w807:refnum<file>, "error out"=w806:errorcluster)  [unwired: 1 in]
        n276 = Close File(refnum=w807, error in=w806) -> (error out=w862:errorcluster)  [unwired: 1 out]
      }
      frame "output-fpp" {
        n277 = local read "FPP - Source"() -> (w959:u32)
        n278 = local read "FPP - Drain"() -> (w960:u32)
        n279 = local read "FPP - Gate"() -> (w961:u32)
        n280 = Number To Decimal String(number=w981) -> (decimal integer string=w1035:string)  [unwired: 1 in]
        n281 = Bundle By Name(cluster=w1011, "Emergency Stop"=w1038) -> (w1048:T1)
        n282 = Delete From Array(array=w1026, index=0 ("Index")) -> (deleted portion=w1024:string, array with subset deleted=w1023:string[])  [unwired: 1 in]
        n283 = VISA Write(VISA resource name=w1002, write buffer=":PAGE:CHAN:MODE SWE;" ("write buffer (\"\")"), error in (no error)=w999) -> (VISA resource name out=w1001:refnum<visa-resource-name>, error out=w1000:errorcluster)  [unwired: 1 out]
        n284 = Concatenate Strings(w1034, "-outputfpp-" ("Substring"), w1035, w980, ".txt" ("Substring")) -> (w1037:string)
        n285 = case shown="\"d\", Default" w1024 {
          tunnel: [w1049 w1050] -> w1022
          frame "s" {
            w1049 = u16 0 items=["Single", "Double"] ("sweep mode")
          }
          frame "d", Default {
            w1050 = u16 1 items=["Single", "Double"] ("sweep mode")
          }
        }
        n286 = Fract/Exp String To Number(string=w1023) -> (number=w1005:dbl[])  [unwired: 3 in, 1 out]
        n287 = String To Path(string=w1037) -> (path=w1033:path)
        n288 = Index Array(array=w1005, index #1=0 ("Index")) -> (element #1=w1021:dbl, element #2=w1020:dbl, element #3=w1019:dbl)  [unwired: 2 in]
        n289 = Delete From Array(array=w1005, length=3 ("Length"), index=0 ("Index")) -> (array with subset deleted=w1004:dbl[])  [unwired: 1 out]
        n290 = local read "FPP - Probe 1"() -> (w957:u32)
        n291 = local read "FPP - Probe 2"() -> (w958:u32)
        n292 = Bundle By Name(cluster=w1013, "Gate Start"=w1021, "Gate Stop"=w1020, "Gate Step (linear only)"=w1019, "Gate Compliance"=w1031, "Range mode"=w997, "Range"=w996) -> (w1047:T6)
        n293 = Index Array(array=w1004, index #1=0 ("Index")) -> (element #1=w1016:dbl, element #2=w1015:dbl, element #3=w1014:dbl)  [unwired: 2 in]
        n294 = call <vilib>:"compatOverwrite.vi"("overwrite (F)"=TRUE) -> ("overwrite?"=w985:T8)
        n295 = Bundle By Name(cluster=w1012, "Drain Start"=w1016, "Drain Stop"=w1015, "Drain Step"=w1014, "Drain Compliance"=w1032, "Range mode"=w995, "Range"=w998) -> (w1046:T7)
        n296 = call "4155C Output-FPP v3.0.vi"("VISA resource name in"=w1001, "FPP - Source"=w959, "Gate"=w1047, "Drain"=w1046, "FPP - Drain"=w960, "Timings"=w1030, "error in (no error)"=w1000, "FPP - Gate"=w961, "FPP - Probe 1"=w957, "sweep mode"=w1022, "FPP - Probe 2"=w958, "Panel controls"=w1048) -> ("VD"=w990:dbl[], "Outparams"=w993:T9, "VISA Resource Name out"=w1028:refnum<visa-resource-name>, "Vprobe2"=w989:dbl[], "ID"=w988:dbl[], "IG"=w987:dbl[], "Vprobe1"=w986:dbl[], "error out"=w1029:errorcluster)  [unwired: 8 in]
        n297 = Unbundle By Name(w993) -> ("V2 Step"=w994:dbl, "V2 Start"=w992:dbl, "Number of points"=w991:i32)
        n298 = Open/Create/Replace File(file path (use dialog)=w1033, error in=w1029, operation (0:open)=w985) -> (refnum out=w1043:refnum<file>, error out=w1044:errorcluster)  [unwired: 3 in, 1 out]
        n299 = call "4155C Make Big 2d array FPP.vi"("1D Var1"=w990, "1d ID"=w988, "1d Vp2"=w989, "1d IG"=w987, "1d Vp1"=w986, "VAR2 START"=w992, "Number of VAR2 steps"=w991, "VAR2 STEP"=w994, "VAR1 Name"="Vd", "Decimal places in header"=i8 1, "VAR2 Name"="Vg") -> ("Header array"=w1039:string[], "Data array"=w1040:dbl[][])  [unwired: 15 in]
        n300 = call "4155C Write array to file.vi"("Byte Stream File Refnum"=w1043, "Header"=w1039, "Data Array"=w1040, "error in (no error)"=w1044) -> ("dup refnum"=w1041:refnum<file>, "error out"=w1042:errorcluster)  [unwired: 1 in]
        n301 = Close File(refnum=w1041, error in=w1042) -> (error out=w1027:errorcluster)  [unwired: 1 out]
      }
      frame "itime" {
        n302 = Delete From Array(array=w1058, index=1) -> (deleted portion=w1057:string)  [unwired: 1 in, 1 out]
        n303 = Delete From Array(array=w1058, index=0 ("Index")) -> (deleted portion=w1086:string)  [unwired: 1 in, 1 out]
        n304 = Fract/Exp String To Number(string=w1057) -> (number=w1056:dbl)  [unwired: 3 in, 1 out]
        n305 = case shown="\"l\"" w1086 {
          tunnel: w1085 -> [w1091 w1093 w1097]
          tunnel: [w1090 w1092 w1096] -> w1078
          tunnel: w1056 -> [w1088 _ w1095]
          frame "s" {
            w1089 = u32 0 items=["short  ", "medium  ", "long  "] ("integration time 2")
            n306 = Bundle By Name(cluster=w1091, "integration time"=w1089, "Short/Long integration time"=w1088) -> (w1090:T4)
          }
          frame "m", Default {
            w1094 = u32 1 items=["short  ", "medium  ", "long  "] ("integration time 2")
            n307 = Bundle By Name(cluster=w1093, "integration time"=w1094) -> (w1092:T4)
          }
          frame "l" {
            w1098 = u32 2 items=["short  ", "medium  ", "long  "] ("integration time 2")
            n308 = Bundle By Name(cluster=w1097, "integration time"=w1098, "Short/Long integration time"=w1095) -> (w1096:T4)
          }
        }
      }
      frame "pulsed" {
        n309 = Delete From Array(array=w1131, index=0 ("Index")) -> (deleted portion=w1132:string, array with subset deleted=w1119:string[])  [unwired: 1 in]
        n310 = case shown="\"on\", Default" w1132 {
          tunnel: w1130 -> [w1142 w1145]
          tunnel: [w1141 w1144] -> w1123
          tunnel: w1119 -> [w1139 _]
          frame "on", Default {
            w1140 = u16 1 items=["Continuous", "Pulsed"] ("sweep method")
            n311 = Fract/Exp String To Number(string=w1139) -> (number=w1137:dbl[])  [unwired: 3 in, 1 out]
            n312 = Index Array(array=w1137, index #1=0 ("Index")) -> (element #1=w1136:dbl, element #2=w1135:dbl, element #3=w1134:dbl)  [unwired: 2 in]
            n313 = Bundle By Name(cluster=w1142, "sweep method"=w1140, "Pulse period"=w1136, "Base voltage"=w1135, "Pulse width"=w1134) -> (w1141:T4)
          }
          frame "off" {
            w1143 = u16 0 items=["Continuous", "Pulsed"] ("sweep method")
            n314 = Bundle By Name(cluster=w1145, "sweep method"=w1143) -> (w1144:T4)
          }
        }
      }
      frame "gaterangemode" {
        n315 = Delete From Array(array=w1176, index=0 ("Index")) -> (deleted portion=w1177:string)  [unwired: 1 in, 1 out]
        n316 = case shown="\"f\"" w1177 {
          tunnel: [w1179 w1180 w1181] -> w1166
          frame "a", Default {
            w1179 = u16 0 items=["Auto", "Limited", "Fixed"] ("Gate Range\nmode 2")
          }
          frame "f" {
            w1180 = u16 2 items=["Auto", "Limited", "Fixed"] ("Gate Range\nmode 2")
          }
          frame "l" {
            w1181 = u16 1 items=["Auto", "Limited", "Fixed"] ("Gate Range\nmode 2")
          }
        }
      }
      frame "gaterange" {
        (unwired) u8 11 items=["10fA  ", "100fA  ", "1nA  ", "10nA", "100nA", "1uA", "10uA", "100uA", "1mA", "10mA", "100mA", "1A"] ("Gate Range 2")
        n317 = Delete From Array(array=w1219, index=0 ("Index")) -> (deleted portion=w1209:string)  [unwired: 1 in, 1 out]
        n318 = Scan Value(string=w1209, format string="") -> (value=w1207:dbl)  [unwired: 1 in, 1 out]
        n319 = Logarithm Base 10(1:w1207) -> (0:w1206:dbl)
        n320 = Round To Nearest(number=w1206) -> (nearest integer value=w1205:dbl)
        n321 = Add(x=w1205, y=11.0) -> (x+y=w1203:dbl)
        n322 = To Unsigned Byte Integer(number=w1203) -> (unsigned 8bit integer=w1202:u8)
      }
      frame "drainrange" {
        (unwired) u8 11 items=["10fA  ", "100fA  ", "1nA  ", "10nA", "100nA", "1uA", "10uA", "100uA", "1mA", "10mA", "100mA", "1A"] ("Gate Range 2")
        n323 = Delete From Array(array=w1258, index=0 ("Index")) -> (deleted portion=w1249:string)  [unwired: 1 in, 1 out]
        n324 = Scan Value(string=w1249, format string="") -> (value=w1247:dbl)  [unwired: 1 in, 1 out]
        n325 = Logarithm Base 10(1:w1247) -> (0:w1246:dbl)
        n326 = Round To Nearest(number=w1246) -> (nearest integer value=w1245:dbl)
        n327 = Add(x=w1245, y=11.0) -> (x+y=w1243:dbl)
        n328 = To Unsigned Byte Integer(number=w1243) -> (unsigned 8bit integer=w1242:u8)
      }
      frame "drainrangemode" {
        n329 = Delete From Array(array=w1290, index=0 ("Index")) -> (deleted portion=w1291:string)  [unwired: 1 in, 1 out]
        n330 = case shown="\"f\"" w1291 {
          tunnel: [w1293 w1294 w1295] -> w1280
          frame "a", Default {
            w1293 = u16 0 items=["Auto", "Limited", "Fixed"] ("Gate Range\nmode 2")
          }
          frame "f" {
            w1294 = u16 2 items=["Auto", "Limited", "Fixed"] ("Gate Range\nmode 2")
          }
          frame "l" {
            w1295 = u16 1 items=["Auto", "Limited", "Fixed"] ("Gate Range\nmode 2")
          }
        }
      }
      frame "Error", Default {
      }
      frame "logfile" {
        n331 = Number To Decimal String(number=w1346) -> (decimal integer string=w1381:string)  [unwired: 1 in]
        n332 = Concatenate Strings(w1380, "logfile" ("Substring"), w1381, w1344, ".txt" ("Substring")) -> (w1378:string)
        n333 = String To Path(string=w1378) -> (path=w1351:path)
        n334 = Unbundle(w1377) -> ("integration time"=w1376:u32, "Short/Long integration time"=w1375:dbl, "hold time (sec)"=w1374:dbl, "delay time (sec)"=w1373:dbl, "Step Time (0 disables)"=w1372:dbl, "sweep method"=w1371:u16, "Pulse period"=w1370:dbl, "Base voltage"=w1369:dbl, "Pulse width"=w1368:dbl)
        n335 = Build Array(w1376, w1375, w1374, w1373, w1372, w1371, w1370, w1369, w1368, w1362, w1363, w1364, w1365, w1366, w1367) -> (w1355:dbl[])
        n336 = Insert Into Array(array=dbl[][] [] ("Input Array"), new element=w1355) -> (w1354:dbl[][])  [unwired: 2 in]
        n337 = call <vilib>:"compatOverwrite.vi"("overwrite (F)"=TRUE) -> ("overwrite?"=w1349:T8)
        n338 = Open/Create/Replace File(file path (use dialog)=w1351, error in=w1353, operation (0:open)=w1349) -> (refnum out=w1359:refnum<file>, error out=w1358:errorcluster)  [unwired: 3 in, 1 out]
        n339 = call "4155C Write array to file.vi"("Byte Stream File Refnum"=w1359, "Header"=string[] ["Int Time", "Short/Long Itime", "Hold time", "Delay time", "Step time", "Sweep method", "Pulse period", "Base Voltage", "Pulse width", "Drain compliance", "Gate compliance", "Gate range mode", "Gate range", "S/D range mode", "S/D range"], "Data Array"=w1354, "error in (no error)"=w1358) -> ("dup refnum"=w1361:refnum<file>, "error out"=w1360:errorcluster)  [unwired: 1 in]
        n340 = Close File(refnum=w1361, error in=w1360) -> (error out=w1352:errorcluster)  [unwired: 1 out]
      }
      frame "sample" {
        w1405 = 1
        # "Add a time offset (elapsed time) to the time axis."
        # "Adjusts graph colors."
        n341 = Number To Decimal String(number=w1437) -> (decimal integer string=w1479:string)  [unwired: 1 in]
        n342 = Fract/Exp String To Number(string=w1476) -> (number=w1441:dbl[])  [unwired: 3 in, 1 out]
        n343 = local read "Sample - Probe 4"() -> (w1387:u32)
        n344 = Concatenate Strings(w1457, "-sample-" ("Substring"), w1479, w1435, ".txt" ("Substring")) -> (w1477:string)
        n345 = local read "Sample - Drain"() -> (w1388:u32)
        n346 = Index Array(array=w1441, index=0 ("Index")) -> (element=w1474:dbl)
        n347 = String To Path(string=w1477) -> (path=w1461:path)
        n348 = Index Array(array=w1441, index=2 ("Index")) -> (element=w1470:dbl)
        n349 = Index Array(array=w1441, index=3 ("Index")) -> (element=w1443:dbl)
        n350 = Index Array(array=w1441, index=4 ("Index")) -> (element=w1440:dbl)
        n351 = Index Array(array=w1441, index=1 ("Index")) -> (element=w1471:dbl)
        n352 = local read "Plot sample extrema vs time"() -> (w1408:bool)
        n353 = local read "Time Units"() -> (w1383:u16)
        n354 = local read "Sample - Gate"() -> (w1390:u32)
        n355 = local read "Sample - Source/Common"() -> (w1389:u32)
        n356 = call "4155C Config Sampling Measurements v3.0.vi"("VISA session"=w1482, "Num Points"=w1470, "Sample - Drain"=w1388, "Display on/off"=TRUE, "Gate Compliance"=w1458, "Sampling interval"=w1440, "Sample - Source/Common"=w1389, "Sample - Probe 4"=w1387, "Drain Compliance"=w1480, "Standby"=w1391, "error in (no error)"=w1481, "Timings"=w1449, "Sample - Gate"=w1390, "Sample time"=w1443) -> ("dup VISA resource name"=w1484:refnum<visa-resource-name>, "error out"=w1483:errorcluster)
        n357 = call "4155C Take Sample v3.0.vi"("VISA resource name in"=w1484, "Emergency Stop"=w1454, "Sample - Gate"=w1390, "Vg"=w1474, "Sample - Drain"=w1388, "Vd"=w1471, "error in (no error)"=w1483) -> ("Time"=w1385:dbl[], "VISA Resource Name out"=w1451:refnum<visa-resource-name>, "Ig"=w1401:dbl[], "Id"=w1402:dbl[], "Is"=w1403:dbl[], "error out"=w1406:errorcluster)  [unwired: 3 in]
        n358 = case shown="0, Default" w1383 {
          tunnel: [w1487 w1488 w1491] -> w1386
          tunnel: w1385 -> [w1486 w1488 w1490]
          frame 2 {
            n359 = Divide(x=w1486, y=3600.0) -> (x/y=w1487:dbl[])
          }
          frame 0, Default {
          }
          frame 1 {
            n360 = Divide(x=w1490, y=60.0) -> (x/y=w1491:dbl[])
          }
        }
        n361 = Insert Into Array(array=w1399, new element=w1402) -> (w1393:dbl[])  [unwired: 1 in]
        n362 = Add(x=w1386, y=w1384) -> (x+y=w1404:dbl[])
        n363 = Insert Into Array(array=w1398, new element=w1403) -> (w1394:dbl[])  [unwired: 1 in]
        n364 = Insert Into Array(array=w1400, new element=w1401) -> (w1396:dbl[])  [unwired: 1 in]
        n365 = case shown="True" w1408 {
          tunnel: w1409 -> [w1492 w1494]
          tunnel: [w1492 w1495] -> w1407
          tunnel: w1404 -> [_ w1493]
          frame False {
          }
          frame True {
            n366 = Insert Into Array(array=w1494, new element=w1493) -> (w1495:i32[])  [unwired: 1 in]
          }
        }
        n367 = case shown="True" "Plot sample extrema vs time" {
          tunnel: w1403 -> [_ w1523]
          tunnel: w1402 -> [_ w1524]
          tunnel: w1401 -> [_ w1525]
          tunnel: [w1502 w1512] -> w1392
          tunnel: w1406 -> [w1502 w1516]
          tunnel: w1430 -> [w1501 w1528]
          tunnel: w1429 -> [w1500 w1527]
          tunnel: w1428 -> [w1499 w1529]
          tunnel: w1427 -> [w1498 w1526]
          tunnel: w1426 -> [w1497 w1531]
          tunnel: w1425 -> [w1496 w1530]
          tunnel: [w1501 w1514] -> w1424
          tunnel: [w1500 w1507] -> w1423
          tunnel: [w1499 w1508] -> w1422
          tunnel: [w1498 w1532] -> w1421
          tunnel: [w1497 w1515] -> w1420
          tunnel: [w1496 w1509] -> w1419
          tunnel: w1407 -> [_ w1503]
          frame False {
          }
          frame True {
            w1510 = 1
            # "Number of VAR2 steps is 1."
            # "abs(Ig)"
            # "abs(Is)"
            # "abs(Id)"
            # "Adjusts graph colors."
            n368 = Absolute Value(x=w1525) -> (abs(x)=w1504:dbl[])
            n369 = Absolute Value(x=w1524) -> (abs(x)=w1505:dbl[])
            n370 = Absolute Value(x=w1523) -> (abs(x)=w1506:dbl[])
            n371 = Array Max & Min(array=w1506) -> (max value=w1522:dbl, min value=w1519:dbl)  [unwired: 2 out]
            n372 = Array Max & Min(array=w1505) -> (max value=w1521:dbl, min value=w1518:dbl)  [unwired: 2 out]
            n373 = Array Max & Min(array=w1504) -> (max value=w1520:dbl, min value=w1517:dbl)  [unwired: 2 out]
            n374 = local write "Id max"(w1521) -> ()
            n375 = local write "Id min"(w1518) -> ()
            n376 = local write "Ig max"(w1520) -> ()
            n377 = local write "Ig min"(w1517) -> ()
            n378 = Insert Into Array(array=w1531, new element=w1504) -> (w1515:dbl[])  [unwired: 1 in]
            n379 = Insert Into Array(array=w1530, new element=w1504) -> (w1509:dbl[])  [unwired: 1 in]
            n380 = local write "Is max"(w1522) -> ()
            n381 = local write "Is min"(w1519) -> ()
            n382 = Insert Into Array(array=w1529, new element=w1505) -> (w1508:dbl[])  [unwired: 1 in]
            n383 = Insert Into Array(array=w1526, new element=w1505) -> (w1532:dbl[])  [unwired: 1 in]
            n384 = Insert Into Array(array=w1528, new element=w1506) -> (w1514:dbl[])  [unwired: 1 in]
            n385 = Insert Into Array(array=w1527, new element=w1506) -> (w1507:dbl[])  [unwired: 1 in]
            n386 = control-ref of="Imax vs time"() -> (w1533:refnum<vi>)
            n387 = call "4155C Config Chart Colours.vi"("Numeric"=w1510, "XY Graph 2"=w1533) -> ()  [unwired: 6 in]
            n388 = call "4155C Split array.vi"("Number of VAR2 steps"=w1510, "Y2 data in"=w1508, "X data in"=w1503, "Y1 data in"=w1514, "Y3 data in"=w1515, "error in (no error)"=w1516) -> ("Array of clusters"=w1534:cluster{"Y data in":dbl[], "X data in":dbl[]}[], "error out"=w1513:errorcluster)  [unwired: 1 in]
            n389 = call "4155C Split array.vi"("Number of VAR2 steps"=w1510, "Y2 data in"=w1508, "X data in"=w1503, "Y1 data in"=w1507, "Y3 data in"=w1509, "error in (no error)"=w1513) -> ("Array of clusters"=w1511:cluster{"Y data in":dbl[], "X data in":dbl[]}[], "error out"=w1512:errorcluster)  [unwired: 1 in]
            n390 = local write "Imax vs time"(w1534) -> ()
            n391 = local write "Imin vs time"(w1511) -> ()
          }
        }
        n392 = Insert Into Array(array=w1397, new element=w1404) -> (w1395:dbl[])  [unwired: 1 in]
        n393 = control-ref of="I vs time (Bias Stress)"() -> (w1412:refnum<vi>)
        n394 = call "4155C Split array.vi"("Number of VAR2 steps"=w1405, "Y2 data in"=w1393, "X data in"=w1395, "Y1 data in"=w1394, "Y3 data in"=w1396) -> ("Array of clusters"=w1411:cluster{"Y data in":dbl[], "X data in":dbl[]}[])  [unwired: 2 in, 1 out]
        n395 = call "4155C Config Chart Colours.vi"("Numeric"=w1405, "XY Graph 2"=w1412) -> ()  [unwired: 6 in]
        n396 = local write "I vs time (Bias Stress)"(w1411) -> ()
        n397 = Insert Into Array(array=dbl[][] [] ("Input Array"), new element=w1404) -> (w1410:dbl[][])  [unwired: 2 in]
        n398 = Insert Into Array(array=w1410, new element=w1401) -> (w1464:dbl[][])  [unwired: 2 in]
        n399 = VISA Write(VISA resource name=w1451, write buffer=":DISP ON" ("write buffer (\"\")"), error in (no error)=w1392) -> (VISA resource name out=w1450:refnum<visa-resource-name>, error out=w1452:errorcluster)  [unwired: 1 out]
        n400 = Insert Into Array(array=w1464, new element=w1402) -> (w1463:dbl[][])  [unwired: 2 in]
        n401 = Insert Into Array(array=w1463, new element=w1403) -> (w1456:dbl[][])  [unwired: 2 in]
        n402 = Transpose 2D Array(2D array=w1456) -> (transposed array=w1455:dbl[][])
        n403 = call <vilib>:"compatOverwrite.vi"("overwrite (F)"=TRUE) -> ("overwrite?"=w1438:T8)
        n404 = Open/Create/Replace File(file path (use dialog)=w1461, error in=w1452, operation (0:open)=w1438) -> (refnum out=w1467:refnum<file>, error out=w1466:errorcluster)  [unwired: 3 in, 1 out]
        n405 = call "4155C Write array to file.vi"("Byte Stream File Refnum"=w1467, "Header"=string[] ["Time /Units", "Ig /A", "Id /A", "Is /A"], "Data Array"=w1455, "error in (no error)"=w1466) -> ("dup refnum"=w1469:refnum<file>, "error out"=w1468:errorcluster)  [unwired: 1 in]
        n406 = Close File(refnum=w1469, error in=w1468) -> (error out=w1459:errorcluster)  [unwired: 1 out]
      }
      frame "samplei" {
        n407 = local read "Sample I - Source/Common"() -> (w1535:u32)
        n408 = Number To Decimal String(number=w1560) -> (decimal integer string=w1611:string)  [unwired: 1 in]
        n409 = local read "Sample I - Probe 4 (Disabled)"() -> (w1538:u32)
        n410 = Concatenate Strings(w1590, "-samplei-" ("Substring"), w1611, w1559, ".txt" ("Substring")) -> (w1609:string)
        n411 = Fract/Exp String To Number(string=w1608) -> (number=w1575:dbl[])  [unwired: 3 in, 1 out]
        n412 = String To Path(string=w1609) -> (path=w1593:path)
        n413 = local read "Sample I - Probe 3 (Disabled)"() -> (w1537:u32)
        n414 = Index Array(array=w1575, index=4 ("Index")) -> (element=w1569:dbl)
        n415 = Index Array(array=w1575, index=3 ("Index")) -> (element=w1570:dbl)
        n416 = Index Array(array=w1575, index=1 ("Index")) -> (element=w1572:dbl)
        n417 = Index Array(array=w1575, index=0 ("Index")) -> (element=w1573:dbl)
        n418 = Index Array(array=w1575, index=2 ("Index")) -> (element=w1571:dbl)
        n419 = local read "Sample I - Drain/Gate"() -> (w1536:u32)
        n420 = call "4155C Config SamplingI Measurements v3.0.vi"("VISA session"=w1614, "Num Points"=w1572, "Sample I - Probe 3 (Disabled)"=w1537, "Display on/off"=TRUE, "Sample I - Source/Common"=w1535, "Sample I - Drain/Gate"=w1536, "Sampling interval"=w1570, "Standby"=w1539, "error in (no error)"=w1613, "Timings"=w1582, "Sample I - Probe 4 (Disabled)"=w1538, "Sample time"=w1571) -> ("dup VISA resource name"=w1616:refnum<visa-resource-name>, "error out"=w1615:errorcluster)  [unwired: 2 in]
        n421 = call "4155C Take SampleI v3.0.vi"("Sample I - Drain/Gate"=w1536, "Emergency Stop"=w1587, "error in (no error)"=w1615, "Idg 2"=w1573, "Vdg compliance 2"=w1569, "VISA resource name in"=w1616) -> ("error out"=w1585:errorcluster, "Idg"=w1618:dbl[], "Vdg"=w1595:dbl[], "VISA Resource Name out"=w1583:refnum<visa-resource-name>, "Is"=w1617:dbl[], "Time"=w1599:dbl[])
        n422 = Insert Into Array(array=dbl[][] [] ("Input Array"), new element=w1599) -> (w1598:dbl[][])  [unwired: 2 in]
        n423 = Insert Into Array(array=w1598, new element=w1595) -> (w1597:dbl[][])  [unwired: 2 in]
        n424 = Insert Into Array(array=w1597, new element=w1618) -> (w1596:dbl[][])  [unwired: 2 in]
        n425 = VISA Write(VISA resource name=w1583, write buffer=":DISP ON" ("write buffer (\"\")"), error in (no error)=w1585) -> (VISA resource name out=w1568:refnum<visa-resource-name>, error out=w1584:errorcluster)  [unwired: 1 out]
        n426 = Insert Into Array(array=w1596, new element=w1617) -> (w1589:dbl[][])  [unwired: 2 in]
        n427 = call <vilib>:"compatOverwrite.vi"("overwrite (F)"=TRUE) -> ("overwrite?"=w1563:T8)
        n428 = Open/Create/Replace File(file path (use dialog)=w1593, error in=w1584, operation (0:open)=w1563) -> (refnum out=w1602:refnum<file>, error out=w1601:errorcluster)  [unwired: 3 in, 1 out]
        n429 = Transpose 2D Array(2D array=w1589) -> (transposed array=w1588:dbl[][])
        n430 = call "4155C Write array to file.vi"("Byte Stream File Refnum"=w1602, "Header"=string[] ["Time /s", "Vdg /V", "Idg /A", "Is /A"], "Data Array"=w1588, "error in (no error)"=w1601) -> ("dup refnum"=w1604:refnum<file>, "error out"=w1603:errorcluster)  [unwired: 1 in]
        n431 = Close File(refnum=w1604, error in=w1603) -> (error out=w1566:errorcluster)  [unwired: 1 out]
        n432 = VISA Write(VISA resource name=w1568, write buffer=";:PAGE:SCON:STAN OFF;:PAGE:CHAN:VSU2:DIS;" ("write buffer (\"\")"), error in (no error)=w1566) -> (VISA resource name out=w1564:refnum<visa-resource-name>, error out=w1565:errorcluster)  [unwired: 1 out]
      }
      frame "#" {
        n433 = VISA Write(VISA resource name=w1643, write buffer=":DISP ON" ("write buffer (\"\")"), error in (no error)=w1642) -> (VISA resource name out=w1641:refnum<visa-resource-name>, error out=w1640:errorcluster)  [unwired: 1 out]
      }
      frame "stressV" {
        n434 = Number To Decimal String(number=w1674) -> (decimal integer string=w1715:string)  [unwired: 1 in]
        n435 = Concatenate Strings(w1699, "-stressV-" ("Substring"), w1715, w1673, ".txt" ("Substring")) -> (w1713:string)
        n436 = Fract/Exp String To Number(string=w1712) -> (number=w1685:dbl[])  [unwired: 3 in, 1 out]
        n437 = local read "Stress V - Drain"() -> (w1652:u32)
        n438 = String To Path(string=w1713) -> (path=w1703:path)
        n439 = Index Array(array=w1685, index=3 ("Index")) -> (element=w1682:dbl)
        n440 = Index Array(array=w1685, index=1 ("Index")) -> (element=w1680:dbl)
        n441 = Index Array(array=w1685, index=0 ("Index")) -> (element=w1679:dbl)
        n442 = Index Array(array=w1685, index=4 ("Index")) -> (element=w1684:dbl)
        n443 = Index Array(array=w1685, index=2 ("Index")) -> (element=w1681:dbl)
        n444 = local read "Stress V - Gate"() -> (w1653:u32)
        n445 = local read "Stress V - Source/Common"() -> (w1654:u32)
        n446 = call "4155C Config V Stress v3.0.vi"("Display on/off"=TRUE, "Stress V - Gate"=w1653, "Stress V - Drain"=w1652, "Stress V - Source/Common"=w1654, "IG compliance"=w1681, "ID compliance"=w1682, "error in (no error)"=w1717, "VG"=w1679, "VD"=w1680, "VISA session"=w1718) -> ("error out"=w1719:errorcluster, "dup VISA resource name"=w1720:refnum<visa-resource-name>)
        n447 = call "4155C Apply Stress.vi"("error in (no error)"=w1719, "Duration"=w1684, "Emergency Stop"=w1698, "VISA resource name in"=w1720) -> ("error out"=w1696:errorcluster, "VISA Resource Name out"=w1694:refnum<visa-resource-name>)
        n448 = VISA Write(VISA resource name=w1694, write buffer=":DISP ON" ("write buffer (\"\")"), error in (no error)=w1696) -> (VISA resource name out=w1693:refnum<visa-resource-name>, error out=w1695:errorcluster)  [unwired: 1 out]
        n449 = call <vilib>:"compatOverwrite.vi"("overwrite (F)"=TRUE) -> ("overwrite?"=w1678:T8)
        n450 = Open/Create/Replace File(file path (use dialog)=w1703, error in=w1695, operation (0:open)=w1678) -> (refnum out=w1706:refnum<file>, error out=w1705:errorcluster)  [unwired: 3 in, 1 out]
        n451 = call "4155C Write array to file.vi"("Byte Stream File Refnum"=w1706, "Header"=string[] ["V stress completed successfully", ""], "error in (no error)"=w1705) -> ("dup refnum"=w1708:refnum<file>, "error out"=w1707:errorcluster)  [unwired: 2 in]
        n452 = Close File(refnum=w1708, error in=w1707) -> (error out=w1701:errorcluster)  [unwired: 1 out]
      }
      frame "stressI" {
        n453 = Number To Decimal String(number=w1742) -> (decimal integer string=w1779:string)  [unwired: 1 in]
        n454 = Concatenate Strings(w1763, "-stressI-" ("Substring"), w1779, w1741, ".txt" ("Substring")) -> (w1777:string)
        n455 = Fract/Exp String To Number(string=w1776) -> (number=w1751:dbl[])  [unwired: 3 in, 1 out]
        n456 = local read "Stress I - Source/Common"() -> (w1721:u32)
        n457 = Index Array(array=w1751, index=1 ("Index")) -> (element=w1747:dbl)
        n458 = Index Array(array=w1751, index=0 ("Index")) -> (element=w1748:dbl)
        n459 = Index Array(array=w1751, index=2 ("Index")) -> (element=w1749:dbl)
        n460 = String To Path(string=w1777) -> (path=w1767:path)
        n461 = local read "Stress I - Drain/Gate"() -> (w1722:u32)
        n462 = call "4155C Config I Stress v3.0.vi"("Stress I - Drain/Gate"=w1722, "Stress I - Source/Common"=w1721, "Display on/off"=TRUE, "error in (no error)"=w1781, "VDG compliance"=w1747, "IDG"=w1748, "VISA session"=w1782) -> ("error out"=w1783:errorcluster, "dup VISA resource name"=w1784:refnum<visa-resource-name>)  [unwired: 1 in]
        n463 = call "4155C Apply Stress.vi"("error in (no error)"=w1783, "Duration"=w1749, "Emergency Stop"=w1762, "VISA resource name in"=w1784) -> ("error out"=w1760:errorcluster, "VISA Resource Name out"=w1758:refnum<visa-resource-name>)
        n464 = VISA Write(VISA resource name=w1758, write buffer=":DISP ON" ("write buffer (\"\")"), error in (no error)=w1760) -> (VISA resource name out=w1757:refnum<visa-resource-name>, error out=w1759:errorcluster)  [unwired: 1 out]
        n465 = call <vilib>:"compatOverwrite.vi"("overwrite (F)"=TRUE) -> ("overwrite?"=w1746:T8)
        n466 = Open/Create/Replace File(file path (use dialog)=w1767, error in=w1759, operation (0:open)=w1746) -> (refnum out=w1770:refnum<file>, error out=w1769:errorcluster)  [unwired: 3 in, 1 out]
        n467 = call "4155C Write array to file.vi"("Byte Stream File Refnum"=w1770, "Header"=string[] ["I stress completed successfully", ""], "error in (no error)"=w1769) -> ("dup refnum"=w1772:refnum<file>, "error out"=w1771:errorcluster)  [unwired: 2 in]
        n468 = Close File(refnum=w1772, error in=w1771) -> (error out=w1765:errorcluster)  [unwired: 1 out]
      }
      frame "vsu2pulse" {
        n469 = Number To Decimal String(number=w1805) -> (decimal integer string=w1840:string)  [unwired: 1 in]
        n470 = Concatenate Strings(w1825, "-vsu2-" ("Substring"), w1840, w1804, ".txt" ("Substring")) -> (w1838:string)
        n471 = Fract/Exp String To Number(string=w1837) -> (number=w1813:dbl[])  [unwired: 3 in, 1 out]
        n472 = String To Path(string=w1838) -> (path=w1829:path)
        n473 = Index Array(array=w1813, index=1 ("Index")) -> (element=w1812:dbl)
        n474 = Index Array(array=w1813, index=0 ("Index")) -> (element=w1810:dbl)
        n475 = local read "VSU2 Stress - Source/Common"() -> (w1785:u32)
        n476 = call "4155C Config VSU2 Stress v3.0.vi"("VISA session"=w1843, "Display on/off"=TRUE, "VSU2"=w1810, "error in (no error)"=w1842, "VSU2 Stress - Source/Common"=w1785) -> ("dup VISA resource name"=w1845:refnum<visa-resource-name>, "error out"=w1844:errorcluster)
        n477 = call "4155C Apply Stress.vi"("error in (no error)"=w1844, "Duration"=w1812, "Emergency Stop"=w1824, "VISA resource name in"=w1845) -> ("error out"=w1822:errorcluster, "VISA Resource Name out"=w1820:refnum<visa-resource-name>)
        n478 = VISA Write(VISA resource name=w1820, write buffer=":DISP ON" ("write buffer (\"\")"), error in (no error)=w1822) -> (VISA resource name out=w1819:refnum<visa-resource-name>, error out=w1821:errorcluster)  [unwired: 1 out]
        n479 = call <vilib>:"compatOverwrite.vi"("overwrite (F)"=TRUE) -> ("overwrite?"=w1809:T8)
        n480 = Open/Create/Replace File(file path (use dialog)=w1829, error in=w1821, operation (0:open)=w1809) -> (refnum out=w1832:refnum<file>, error out=w1831:errorcluster)  [unwired: 3 in, 1 out]
        n481 = call "4155C Write array to file.vi"("Byte Stream File Refnum"=w1832, "Header"=string[] ["VSU2 pulse completed successfully", ""], "error in (no error)"=w1831) -> ("dup refnum"=w1834:refnum<file>, "error out"=w1833:errorcluster)  [unwired: 2 in]
        n482 = Close File(refnum=w1834, error in=w1833) -> (error out=w1827:errorcluster)  [unwired: 1 out]
      }
      frame "sample-fpp" {
        w1881 = string[] ["Time /s", "Id VgVd /A", "Ig VgVd /A", "Vp1 VgVd /V", "Vp2 VgVd /V"] ("Header")
        w1885 = "%d" ("format string")
        n483 = local read "FPP - Drain"() -> (w1847:u32)
        n484 = local read "FPP - Source"() -> (w1846:u32)
        n485 = Fract/Exp String To Number(string=w1930) -> (number=w1918:dbl[])  [unwired: 3 in, 1 out]
        n486 = local read "FPP - Probe 1"() -> (w1850:u32)
        n487 = Number To Decimal String(number=w1871) -> (decimal integer string=w1933:string)  [unwired: 1 in]
        n488 = Concatenate Strings(w1924, "-samplefpp-" ("Substring"), w1933, w1870, ".txt" ("Substring")) -> (w1931:string)
        n489 = local read "FPP - Gate"() -> (w1848:u32)
        n490 = String To Path(string=w1931) -> (path=w1893:path)
        n491 = local read "FPP - Probe 2"() -> (w1849:u32)
        n492 = Index Array(array=w1918, index=0 ("Index")) -> (element=w1880:dbl)
        n493 = Index Array(array=w1918, index=1 ("Index")) -> (element=w1879:dbl)
        n494 = Index Array(array=w1918, index=2 ("Index")) -> (element=w1926:dbl)
        n495 = Index Array(array=w1918, index=3 ("Index")) -> (element=w1916:dbl)
        n496 = call "4155C Config Sampling Measurements FPP v3.0.vi"("VISA session"=w1936, "Gate Compliance"=w1925, "FPP - Source"=w1846, "FPP - Drain"=w1847, "Drain Compliance"=w1934, "error in (no error)"=w1935, "Num Points"=w1926, "Timings"=w1923, "FPP - Gate"=w1848, "FPP - Probe 1"=w1850, "Vg"=w1880, "Vd"=w1879, "Display on/off"=TRUE, "Sample time"=w1916, "FPP - Probe 2"=w1849, "Standby"=w1851) -> ("dup VISA resource name"=w1895:refnum<visa-resource-name>, "error out"=w1894:errorcluster)  [unwired: 2 in]
        n497 = Number To Decimal String(number=w1880) -> (decimal integer string=w1905:string)  [unwired: 1 in]
        n498 = call "4155C Take Sample FPP.vi"("VISA resource name in"=w1895, "error in (no error)"=w1894, "Emergency Stop"=w1896) -> ("Time"=w1900:dbl[], "Vp1"=w1910:dbl[], "VISA Resource Name out"=w1877:refnum<visa-resource-name>, "Ig"=w1898:dbl[], "Id"=w1899:dbl[], "Vp2"=w1908:dbl[], "error out"=w1897:errorcluster)  [unwired: 10 in]
        n499 = Insert Into Array(array=dbl[][] [] ("Input Array"), new element=w1900) -> (w1914:dbl[][])  [unwired: 2 in]
        n500 = Number To Decimal String(number=w1879) -> (decimal integer string=w1903:string)  [unwired: 1 in]
        n501 = Insert Into Array(array=w1914, new element=w1899) -> (w1913:dbl[][])  [unwired: 2 in]
        n502 = Concatenate Strings("(Vg = " ("Substring"), w1905, "V, Vd = " ("Substring"), w1903, "V)" ("Substring")) -> (w1901:string)
        n503 = Insert Into Array(array=w1913, new element=w1898) -> (w1912:dbl[][])  [unwired: 2 in]
        n504 = Insert Into Array(array=w1912, new element=w1910) -> (w1909:dbl[][])  [unwired: 2 in]
        n505 = Insert Into Array(array=w1909, new element=w1908) -> (w1878:dbl[][])  [unwired: 2 in]
        n506 = Transpose 2D Array(2D array=w1878) -> (transposed array=w1907:dbl[][])
        n507 = call <vilib>:"compatOverwrite.vi"("overwrite (F)"=TRUE) -> ("overwrite?"=w1875:T8)
        n508 = Open/Create/Replace File(file path (use dialog)=w1893, error in=w1897, operation (0:open)=w1875) -> (refnum out=w1890:refnum<file>, error out=w1891:errorcluster)  [unwired: 3 in, 1 out]
        n509 = Array To Spreadsheet String(array=w1881, 3:w1885) -> (spreadsheet string=w1887:string)  [unwired: 1 in]
        n510 = Search and Replace String(replace all?=TRUE ("replace all? (F)"), input string=w1887, search string="VgVd", replace string=w1901) -> (result string=w1883:string)  [unwired: 4 in, 3 out]
        n511 = Spreadsheet String To Array(format string=w1885, spreadsheet string=w1883, array type (2D Dbl)=w1881) -> (array=w1882:string[])  [unwired: 1 in]
        n512 = call "4155C Write array to file.vi"("Byte Stream File Refnum"=w1890, "Header"=w1882, "Data Array"=w1907, "error in (no error)"=w1891) -> ("dup refnum"=w1888:refnum<file>, "error out"=w1889:errorcluster)  [unwired: 1 in]
        n513 = Close File(refnum=w1888, error in=w1889) -> (error out=w1876:errorcluster)  [unwired: 1 out]
      }
      frame "resample-fpp" {
        w1969 = string[] ["Time /s", "Id VgVd /A", "Ig VgVd /A", "Vp1 VgVd /V", "Vp2 VgVd /V"] ("Header")
        w1973 = "%d" ("format string")
        n514 = Number To Decimal String(number=w1955) -> (decimal integer string=w2013:string)  [unwired: 1 in]
        n515 = Fract/Exp String To Number(string=w2010) -> (number=w1962:dbl[])  [unwired: 3 in, 1 out]
        n516 = Concatenate Strings(w2006, "-resamplefpp-" ("Substring"), w2013, w1956, ".txt" ("Substring")) -> (w2011:string)
        n517 = String To Path(string=w2011) -> (path=w1981:path)
        n518 = Index Array(array=w1962, index=0 ("Index")) -> (element=w1968:dbl)
        n519 = Index Array(array=w1962, index=1 ("Index")) -> (element=w1967:dbl)
        n520 = Number To Decimal String(number=w1968) -> (decimal integer string=w1991:string)  [unwired: 1 in]
        n521 = call "4155C Take Sample FPP.vi"("VISA resource name in"=w1964, "error in (no error)"=w1963, "Emergency Stop"=w1982) -> ("Time"=w1986:dbl[], "Vp1"=w1996:dbl[], "VISA Resource Name out"=w1966:refnum<visa-resource-name>, "Ig"=w1984:dbl[], "Id"=w1985:dbl[], "Vp2"=w1994:dbl[], "error out"=w1983:errorcluster)  [unwired: 10 in]
        n522 = Insert Into Array(array=dbl[][] [] ("Input Array"), new element=w1986) -> (w2000:dbl[][])  [unwired: 2 in]
        n523 = Number To Decimal String(number=w1967) -> (decimal integer string=w1989:string)  [unwired: 1 in]
        n524 = Insert Into Array(array=w2000, new element=w1985) -> (w1999:dbl[][])  [unwired: 2 in]
        n525 = Concatenate Strings("(Vg = " ("Substring"), w1991, "V, Vd = " ("Substring"), w1989, "V)" ("Substring")) -> (w1987:string)
        n526 = Insert Into Array(array=w1999, new element=w1984) -> (w1998:dbl[][])  [unwired: 2 in]
        n527 = Insert Into Array(array=w1998, new element=w1996) -> (w1995:dbl[][])  [unwired: 2 in]
        n528 = Insert Into Array(array=w1995, new element=w1994) -> (w1961:dbl[][])  [unwired: 2 in]
        n529 = call <vilib>:"compatOverwrite.vi"("overwrite (F)"=TRUE) -> ("overwrite?"=w1960:T8)
        n530 = Open/Create/Replace File(file path (use dialog)=w1981, error in=w1983, operation (0:open)=w1960) -> (refnum out=w1978:refnum<file>, error out=w1979:errorcluster)  [unwired: 3 in, 1 out]
        n531 = Array To Spreadsheet String(array=w1969, 3:w1973) -> (spreadsheet string=w1975:string)  [unwired: 1 in]
        n532 = Transpose 2D Array(2D array=w1961) -> (transposed array=w1993:dbl[][])
        n533 = Search and Replace String(replace all?=TRUE ("replace all? (F)"), input string=w1975, search string="VgVd", replace string=w1987) -> (result string=w1971:string)  [unwired: 4 in, 3 out]
        n534 = Spreadsheet String To Array(format string=w1973, spreadsheet string=w1971, array type (2D Dbl)=w1969) -> (array=w1970:string[])  [unwired: 1 in]
        n535 = call "4155C Write array to file.vi"("Byte Stream File Refnum"=w1978, "Header"=w1970, "Data Array"=w1993, "error in (no error)"=w1979) -> ("dup refnum"=w1976:refnum<file>, "error out"=w1977:errorcluster)  [unwired: 1 in]
        n536 = Close File(refnum=w1976, error in=w1977) -> (error out=w1965:errorcluster)  [unwired: 1 out]
      }
      frame "serial" {
        n537 = local read "Termination char\n(0xA = '\\n' = LF)\n(0xD = '\\r' = CR)"() -> (w2040:u8)
        n538 = local read "Enable Termination\nChar (T)"() -> (w2041:bool)
        n539 = Index Array(array=w2048, index=0 ("Index")) -> (element=w2047:string)
        n540 = local read "parity"() -> (w2031:u16)
        n541 = local read "Delay before read (ms)"() -> (w2042:u32)
        n542 = local read "byte count"() -> (w2039:u32)
        n543 = local read "VISA resource name"() -> (w2035:refnum<visa-resource-name>)
        n544 = local read "baud rate"() -> (w2034:u32)
        n545 = local read "Serial End Mode for Reads"() -> (w2033:u16)
        n546 = local read "Timeout (ms)"() -> (w2038:u32)
        n547 = local read "data bits"() -> (w2032:u16)
        n548 = local read "stop bits"() -> (w2037:u16)
        n549 = local read "flow control"() -> (w2036:u16)
        n550 = call "Serial write and read v0.5.vi"("Delay before read (ms)"=w2042, "Termination char\n(0xA = '\\n' = LF)\n(0xD = '\\r' = CR)"=w2040, "Enable Termination\nChar (T)"=w2041, "parity"=w2031, "stop bits"=w2037, "string to write"=w2047, "flow control"=w2036, "byte count"=w2039, "Serial Settings:Serial End Mode for Reads"=w2033, "Timeout (ms)"=w2038, "error in (no error)"=w2053, "VISA resource name"=w2035, "baud rate"=w2034, "data bits"=w2032) -> ("Serial port output"=w2043:string, "error out"=w2052:errorcluster)
        n551 = Build Array (concatenate)(w2043, w2044) -> (w2045:string[])
      }
    }
    "Probe 4 Indicator" <- w61
    "Timings Indicator" <- w62
    n552 = local read "Time Units"() -> (w95:u16)
    n553 = case shown="0" w95 {
      tunnel: ["Time (Seconds)" ("element") "Time (Minutes)" ("element") "Time (Hours)" ("element")] -> w64
      frame 0 {
      }
      frame 1, Default {
      }
      frame 2 {
      }
    }
    n554 = Build Array(w144, w101, w111, w110, w109, w108, w107, w106, w105, w104, w103, w102, w100) -> (w165:dbl[][])
    n555 = Transpose 2D Array(2D array=w165) -> (transposed array=w164:dbl[][])
    n556 = Concatenate Strings(w70, "-I-vs-time.txt" ("Suffix (Imax,Imin,Ion,Ioff)")) -> (w175:string)
    n557 = Build Array(w64, "Is max (A)" ("VAR2 Name"), "Is min (A)" ("VAR2 Name"), "Id max (A)" ("VAR2 Name"), "Id min (A)" ("VAR2 Name"), "Ig max (A)" ("VAR2 Name"), "Ig min (A)" ("VAR2 Name"), "Is on (A)" ("VAR2 Name"), "Is off (A)" ("VAR2 Name"), "Id on (A)" ("VAR2 Name"), "Id off (A)" ("VAR2 Name"), "Ig on (A)" ("VAR2 Name"), "Ig off (A)" ("VAR2 Name")) -> (w170:string[])
    n558 = Array To Spreadsheet String(array=w164, 3:"%e" ("format string")) -> (spreadsheet string=w168:string)  [unwired: 1 in]
    n559 = Array To Spreadsheet String(array=w170, 3:"" ("format string")) -> (spreadsheet string=w169:string)  [unwired: 1 in]
    n560 = String To Path(string=w175) -> (path=w174:path)
    n561 = Build Array(w169, w168) -> (w167:string[])
    n562 = Write to Text File(file (use dialog)=w174, text=w167, error in=w143) -> (refnum out=w176:refnum<file>, error out=w166:errorcluster)  [unwired: 1 in, 1 out]
    n563 = Close File(refnum=w176, error in=w166) -> (error out=w98:errorcluster)  [unwired: 1 out]
    n564 = Concatenate Strings(w70, "-serial-port.txt" ("Suffix (serial port log)")) -> (w146:string)
    n565 = String To Path(string=w146) -> (path=w145:path)
    n566 = Build Array(w64, "Serial port input" ("VAR2 Name"), "Serial port output: ") -> (w136:string[])
    n567 = Array To Spreadsheet String(array=w140, 3:"" ("format string")) -> (spreadsheet string=w133:string)  [unwired: 1 in]
    n568 = Array To Spreadsheet String(array=w136, 3:"" ("format string")) -> (spreadsheet string=w134:string)  [unwired: 1 in]
    n569 = Build Array(w134, w133) -> (w135:string[])
    n570 = Array To Spreadsheet String(array=w139, 3:"" ("format string")) -> (spreadsheet string=w151:string)  [unwired: 1 in]
    n571 = Write to Text File(file (use dialog)=w145, text=w135, error in=w98) -> (refnum out=w147:refnum<file>, error out=w148:errorcluster)  [unwired: 1 in, 1 out]
    n572 = Close File(refnum=w147, error in=w148) -> (error out=w71:errorcluster)  [unwired: 1 out]
    n573 = local write "Serial port data"(w151) -> ()
    n574 = Build Array(w69, w68, w67, w66) -> (w80:dbl[][])
    n575 = Build Array(w64, "Is (A)" ("VAR2 Name"), "Id (A)" ("VAR2 Name"), "Ig (A)" ("VAR2 Name")) -> (w76:string[])
    n576 = Transpose 2D Array(2D array=w80) -> (transposed array=w79:dbl[][])
    n577 = Concatenate Strings(w70, "-sample.txt" ("Suffix (Imax,Imin,Ion,Ioff)")) -> (w86:string)
    n578 = Array To Spreadsheet String(array=w76, 3:"" ("format string")) -> (spreadsheet string=w75:string)  [unwired: 1 in]
    n579 = Array To Spreadsheet String(array=w79, 3:"%e" ("format string")) -> (spreadsheet string=w83:string)  [unwired: 1 in]
    n580 = String To Path(string=w86) -> (path=w85:path)
    n581 = Build Array(w75, w83) -> (w82:string[])
    n582 = Write to Text File(file (use dialog)=w85, text=w82, error in=w71) -> (refnum out=w87:refnum<file>, error out=w81:errorcluster)  [unwired: 1 in, 1 out]
    n583 = Close File(refnum=w87, error in=w81) -> (error out=w63:errorcluster)  [unwired: 1 out]
    "error out" <- w63
  }
  "Is max" <- w12
  "Id max" <- w12
  "Ig max" <- w12
  "Imax vs time" <- w2
  "I vs Vg" <- w2
  "Imin vs time" <- w2
  "I vs Vd" <- w2
  "Serial port data" <- "" ("Serial port data")
  "Is min" <- w11
  "Id min" <- w11
  "Ig min" <- w11
  "Ion vs time" <- w2
  "Ioff vs time" <- w2
  "Is on" <- w10
  "Id on" <- w10
  "Ig on" <- w10
  "Is off" <- w9
  "Id off" <- w9
  "Ig off" <- w9
  "I vs time (Bias Stress)" <- w2
